vi "BStAT_(Singles).vi"() -> ()   [LabVIEW 2013]
uses:
  <vilib>/Utility/file.llb/Read From Spreadsheet File (DBL).vi
  <vilib>/Utility/file.llb/Write To Spreadsheet File (I64).vi
panel:
  out "framesPerSecond":u32
  out "serve to point":dbl[](array[numeric])
  in  "Word._Application":refnum<k7>
  out "p2y":dbl[](array[numeric])
  out "p1y":dbl[](array[numeric])
  out "point frames":dbl[](array[numeric])
  out "service frames":dbl[](array[numeric])
  out "comp_p1 2":dbl[](array[numeric])
  out "comp_p2 2":dbl[](array[numeric])
  out "comp_p2":dbl[](array[numeric])
  out "comp_p1":dbl[](array[numeric])
  out "game":i32[][](array[numeric])
  out "save2_data":dbl[][](array[numeric])
  out "save1_data":dbl[][](array[numeric])
  out "save2":i32[][](array[numeric])
  out "save1":i32[][](array[numeric])
  out "filedata in":dbl[][](array[numeric]) format="%0.3f"
  out "edited\nevents":dbl[][](array[numeric])
  out "edited to play":dbl[](array[numeric])
  out "P2 position":bool
  out "P1 position":bool
  out "p2code":i32
  out "p1code":i32
  out "frames":dbl[](array[numeric])
  out "Events":bool[](array[boolean])
  out "coded data":dbl[][](array[numeric])
  out "frame data":dbl[][](array[numeric])
  out "Score":dbl[][](array[numeric])
  out "OH":bool[](array[boolean])
  out "BH":bool[](array[boolean])
  out "FH":bool[](array[boolean])
  in  "stop":bool
  in  "Tab Control":enum32{"Coding", "Display"}(tab)
  in  "switch sides":bool
  in  "Drag control":u32(slide) min=400 max=3000 scale=0.0..6657.0
  in  "UNDO":bool
  out "Last coded":i32
  in  "Progress...":i32(slide) min=400 max=3000 scale=0.0..6657.0
  in  "1":bool
  in  "E2":bool
  in  "E1":bool
  in  "P2":i32
  in  "W2":bool
  in  "W1":bool
  in  "P1":i32
  in  "Pause 2":bool
  in  "F_Fr":bool
  in  "S_Fr":bool
  out "Video":T1(plugin-control)
  in  "START":bool
  in  "Video file":path caption="Open AVI file"
  in  "Save data":path caption="Save data to file"
  in  "Start Coding":bool
  out "F_frame":u32
  out "S_frame":u32
  in  "playback speed":dbl(slide) step=0.25 scale=0.25..2.0
  in  "fast forward":bool
  in  "TL 2":bool
  in  "BR 2":bool
  in  "BL 2":bool
  in  "BC 2":bool
  in  "MR  2":bool
  in  "MC 2":bool
  in  "ML 2":bool
  in  "TR 2":bool
  in  "TC 2":bool
  in  "TL 3":bool
  in  "BR 3":bool
  in  "BL 3":bool
  in  "BC 3":bool
  in  "MR  3":bool
  in  "MC 3":bool
  in  "ML 3":bool
  in  "TR 3":bool
  in  "TC 3":bool
  in  "Pause 1":bool
  out "coding":i32[][](array[numeric])
  in  "1 6":bool
  in  "2 6":bool
  in  "3 6":bool
  in  "4 6":bool
  in  "5 6":bool
  in  "6 6":bool
  in  "7 6":bool
  in  "8 6":bool
  in  "1 5":bool
  in  "2 5":bool
  in  "3 5":bool
  in  "4 5":bool
  in  "5 5":bool
  in  "6 5":bool
  in  "7 5":bool
  in  "8 5":bool
  in  "8 3":bool
  in  "7 3":bool
  in  "6 3":bool
  in  "5 3":bool
  in  "4 3":bool
  in  "3 3":bool
  in  "2 3":bool
  in  "1 3":bool
  in  "8 4":bool
  in  "7 4":bool
  in  "6 4":bool
  in  "5 4":bool
  in  "4 4":bool
  in  "3 4":bool
  in  "2 4":bool
  in  "1 4":bool
  in  "1 2":bool
  in  "2 2":bool
  in  "3 2":bool
  in  "4 2":bool
  in  "5 2":bool
  in  "6 2":bool
  in  "7 2":bool
  in  "8 2":bool
  in  "5":bool
  in  "6":bool
  in  "7":bool
  in  "8":bool
  in  "1":bool
  in  "2":bool
  in  "3":bool
  in  "4":bool
  in  "S2":bool
  in  "S1":bool
  in  "2":bool
  in  "3":bool
  in  "4":bool
  in  "Pause 3":bool
  in  "Stop and save":bool
  out "Numeric":dbl format="%<%H:%M:%S>t"
  in  "play back":i32(slide)=1 min=0 max=5284 scale=0.0..5284.0
  out "DISP":T1(plugin-control)
  in  "Vid file":path caption="Open AVI file"
  in  "Data file":path caption="Read data from"
  in  "Tab Control 2":enum32{"Edit ", "Data Display", "Momentum"}(tab)
  in  "shots":u8(slide)=2 scale=0.0..5.0
  in  "point 2":bool
  in  "Rally":bool
  in  "Write VI":path caption="Write to AVI file"
  in  "before":u8(slide)=2
  in  "Playback Speed":dbl(slide)=1.0 min=0.25 max=30.0 step=0.25 scale=0.25..2.0
  in  "pause":bool
  in  "stop 2":bool
  in  "Playback\nscore":bool
  in  "P2 score":dbl
  in  "P1 score":dbl
  in  "error":bool
  in  "winner":bool
  in  "point 1":bool
  in  "player1":bool
  in  "player2":bool
  in  "1 7":bool
  in  "service2":bool
  in  "service1":bool
  in  "2 7":bool
  in  "3 7":bool
  in  "4 7":bool
  in  "TL":bool
  in  "BR":bool
  in  "BL":bool
  in  "BM":bool
  in  "CR":bool
  in  "CM":bool
  in  "CL":bool
  in  "TR":bool
  in  "TM":bool
  in  "FH 2":bool
  in  "BH 2":bool
  in  "ST":bool
  in  "CR 2":bool
  in  "lob":bool
  in  "clear":bool
  in  "drive":bool
  in  "smash":bool
  in  "defense":bool
  in  "chop":bool
  in  "drop":bool
  in  "net":bool
  in  "OH 2":bool
  in  "Play":bool
  in  "after":u8(slide)=2 scale=0.0..5.0
  in  "write file":bool
  out "Search events":i32(slide) caption="Scaning(events)..." min=400 max=3000 scale=0.0..425.0
  out "Search score":i32(slide) caption="Searching(score)..." min=400 max=3000 scale=0.0..389.0
  out "writing":i32(slide) caption="Writing..." min=400 max=3000 scale=0.0..5284.0
  in  "3 shots":bool
  in  "Compare":bool
  in  "2":string(combo)="1"
  in  "1":string(combo)="1"
  in  "save2":string
  in  "save1":string
  in  "save2":bool
  in  "save1":bool
  in  "Percentage":bool
  in  "display\nselection":string(combo)="1"
  in  "To make white":enum32{""}(tab)
  out "player1 2":string[](array[string])
  out "player2 2":string[](array[string])
  out "P1graph":cluster{dbl[], "array":dbl[]}(graph)={[0.0, nan, 0.0, nan, 0.0, nan, 0.0, nan, 0.0, nan, 0.0, nan, 0.0, nan, 0.0, nan, 0.0], "array"=[1.0, 2.0, 3.0, 4.0, 5.0, 6.0, 7.0, 8.0, 9.0, 10.0, 11.0, 12.0, 13.0, 14.0, 15.0, 16.0, 17.0]}
  out "P2graph":cluster{dbl[], "array":dbl[]}(graph)={[0.0, nan, 0.0, nan, 0.0, nan, 0.0, nan, 0.0, nan, 0.0, nan, 0.0, nan, 0.0, nan, 0.0], "array"=[1.0, 2.0, 3.0, 4.0, 5.0, 6.0, 7.0, 8.0, 9.0, 10.0, 11.0, 12.0, 13.0, 14.0, 15.0, 16.0, 17.0]}
  out "W1/E1":string[](array[string])
  out "W2/E2":string[](array[string])
  out "W/E2":string[](array[string])=["Fore hand", "Back hand", "Over head", "", "Strainght", "Cross", "", "Lob", "Clear", "Drive", "Smash", "Defence", "Chop", "Drop", "Net"]
  out "W/E1":string[](array[string])=["Fore hand", "Back hand", "Over head", "", "Strainght", "Cross", "", "Lob", "Clear", "Drive", "Smash", "Defence", "Chop", "Drop", "Net"]
  out "player2_2":string[](array[string])
  out "player1_2":string[](array[string])
  out "Player 2":string[](array[string])=["Fore hand", "Back hand", "Over head", "", "Straight", "Cross", "", "Smash", "Defense", "Drive/Tap", "Lob", "Drop", "Chop", "Clear", "Net"]
  out "Player 2_2":string[](array[string])=["Fore hand", "Back hand", "Over head", "", "Strainght", "Cross", "", "Lob", "Clear", "Drive", "Smash", "Defence", "Chop", "Drop", "Net"]
  out "Player 1_2":string[](array[string])=["Fore hand", "Back hand", "Over head", "", "Strainght", "Cross", "", "Lob", "Clear", "Drive", "Smash", "Defence", "Chop", "Drop", "Net"]
  out "Player 1":string[](array[string])=["Fore hand", "Back hand", "Over head", "", "Straight", "Cross", "", "Smash", "Defense", "Drive/Tap", "Lob", "Drop", "Chop", "Clear", "Net"]
  out "p2 17":string
  out "p2 16":string
  out "p2 11":string
  out "p2 10":string
  out "p2 9":string
  out "p2 14":string
  out "p2 13":string
  out "p2 12":string
  out "p2 15":string
  out "p1 5":string
  out "p1 7":string
  out "p1 6":string
  out "p1 4":string
  out "p1 1":string
  out "p1 3":string
  out "p1 2":string
  out "p1 8":string
  out "p1 9":string
  in  "to make white 2":enum32{""}(tab)
  out "Shortest rally length(sec)":dbl format="%#_3g"
  out "Longest rally length(sec)":dbl format="%#_3g"
  out "momentum graph":cluster{dbl[], dbl[]}[](graph)
  out "Score":dbl[](array[numeric])
  out "Average rally length(sec)":dbl format="%#_3g"
  out "Rally length(sec)":dbl format="%#_3g"
  in  "edit video":bool
  in  "REPORT":bool
  # "Strategic Analysis Tool for Badminton"
  # "Forehand"
  # "Backhand"
  # "Overhead"
  # "Position"
  # "Straight"
  # "Cross"
  # "Straight"
  # "Cross"
  # "Straight"
  # "Cross"
  # "Smash"
  # "Defence"
  # "Drive/Tap"
  # "Lob"
  # "Drop"
  # "Chop"
  # "Clear"
  # "Net"
  # "Score"
  # "© 2014 National Sports Institute of Malaysia All Rights Reserved"
  # "© 2012 National Sports Institute of Malaysia All Rights Reserved"
  # "Shots to Playback"
  # "Score"
  # "Player"
  # "Position"
  # "Special Events"
  # "Playback interval (s)"
  # "to"
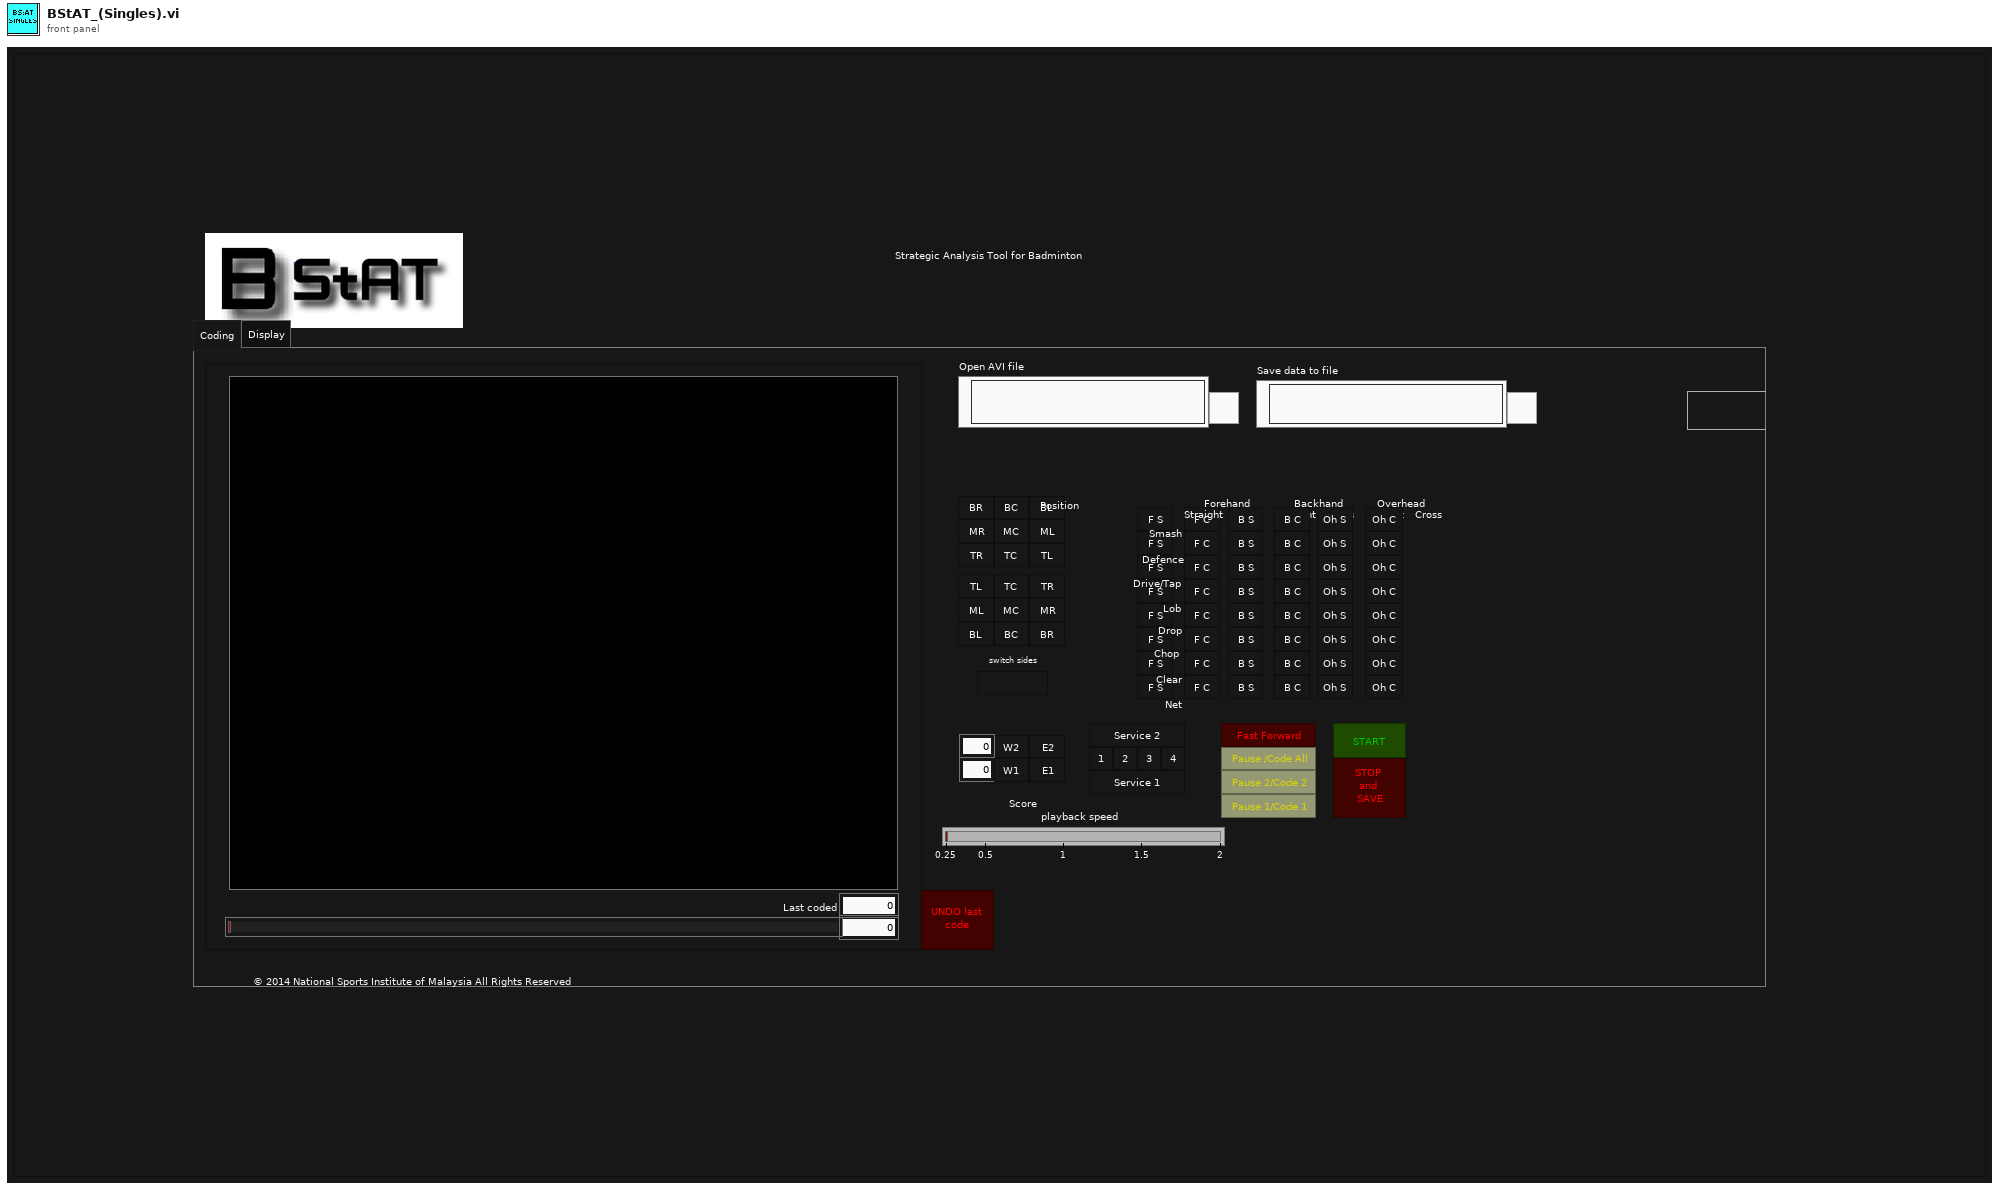
[diagram p1: front panel]
types:
  T1 = typedef "IMAQ Image.ctl" = refnum<image>
  T2 = enum8{"Enabled", "Disabled", "Disabled and Grayed Out"}
  T3 = enum16{"open", "replace", "create", "open or create", "replace or create", "replace or create with confirmation"}
  T4 = typedef "Image Type" = u32
  T5 = typedef "AviRefnum.ctl" = refnum<k1>
  T6 = cluster{"width":u32, "height":u32, "framesPerSecond":u32, "compressionFilter":string, "hasData":bool}
  T7 = typedef "LVPositionTypeDef.ctl" = cluster{"Left":i32, "Top":i32}
  T8 = cluster{"Position":T7, "Position":T7, "Position":T7, "Position":T7, "Position":T7, "Position":T7, "Position":T7, "Position":T7, "Position":T7, "Position":T7}
  T9 = cluster{"Position":T7, "Position":T7, "Position":T7, "Position":T7, "Position":T7, "Position":T7}
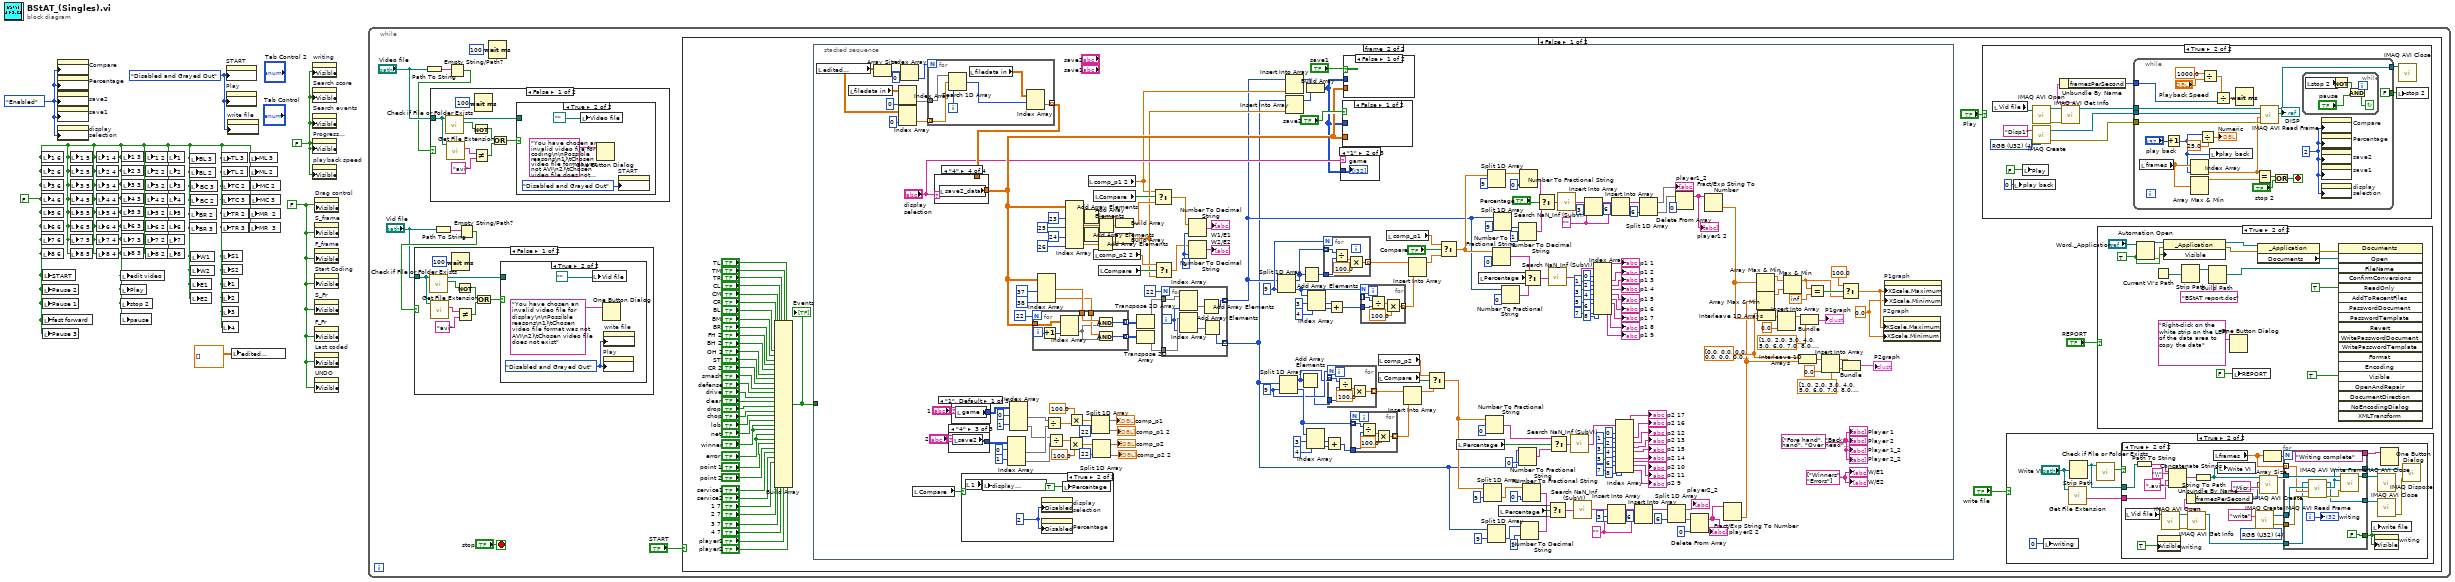
[diagram p0: block diagram]
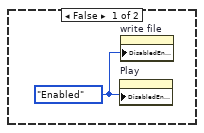
[diagram p2: hidden frame]
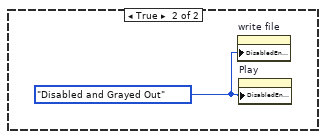
[diagram p3: hidden frame]
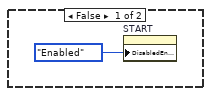
[diagram p4: hidden frame]
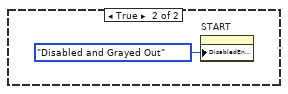
[diagram p5: hidden frame]
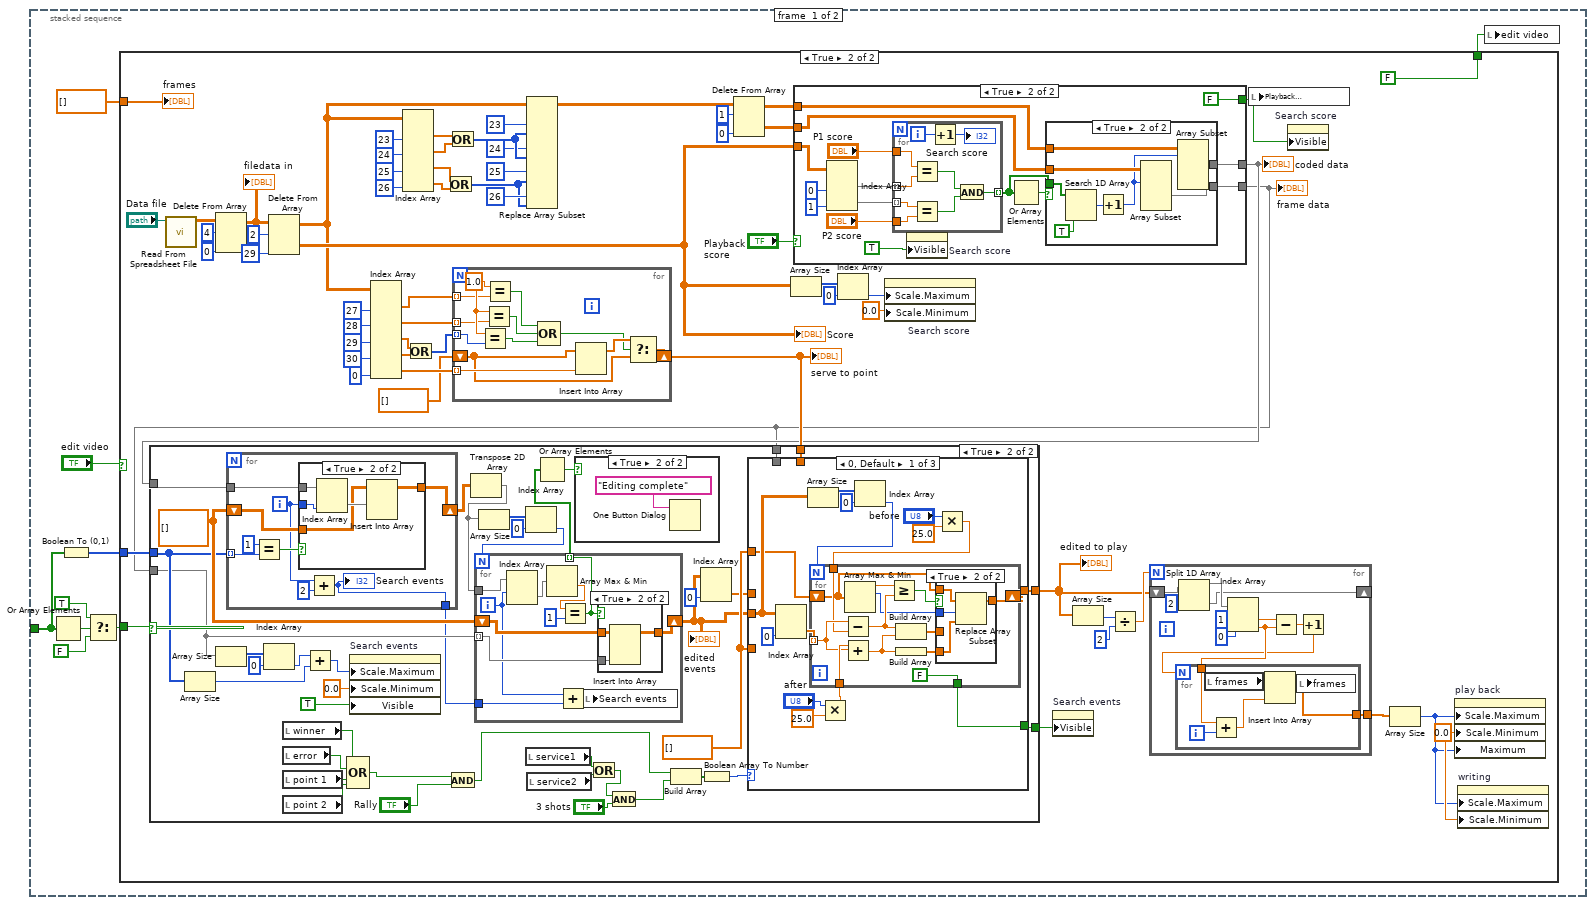
[diagram p7: hidden frame]
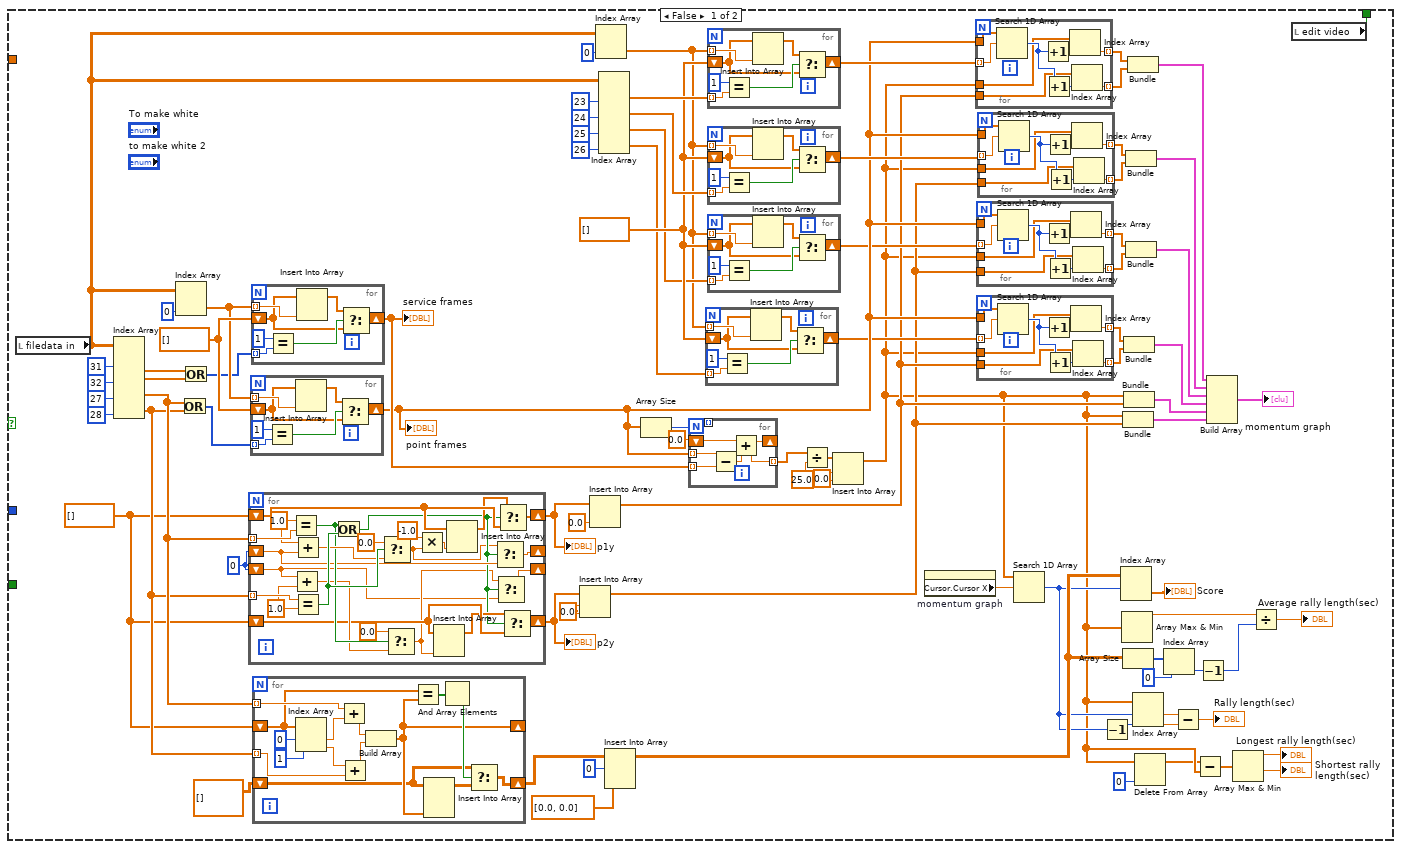
[diagram p8: hidden frame]
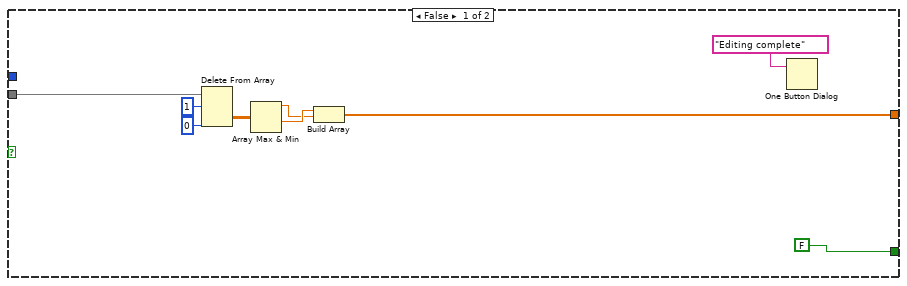
[diagram p9: hidden frame]
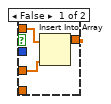
[diagram p10: hidden frame]
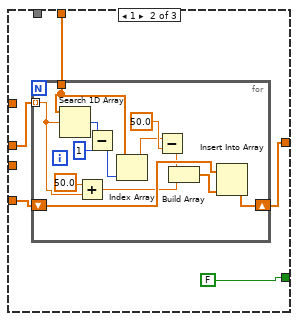
[diagram p11: hidden frame]
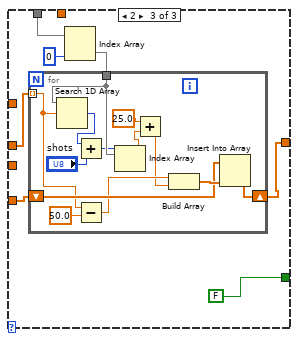
[diagram p12: hidden frame]
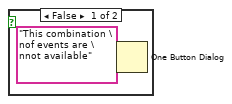
[diagram p13: hidden frame]
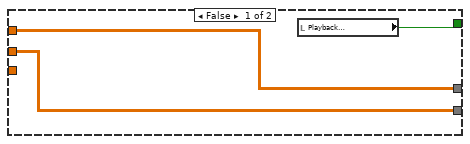
[diagram p16: hidden frame]
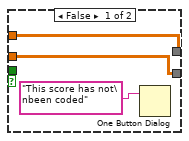
[diagram p17: hidden frame]
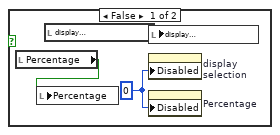
[diagram p18: hidden frame]
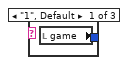
[diagram p19: hidden frame]
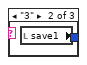
[diagram p20: hidden frame]
diagram:
  w1 = T2."Enabled" ("Disabled")
  w2 = T2."Disabled and Grayed Out" ("Disabled")
  w4 = FALSE ("4 6")
  w3 = FALSE ("Visible")
  w5 = FALSE ("Visible")
  n1 = local write "1 6"(w4) -> ()
  n2 = local write "2 6"(w4) -> ()
  n3 = local write "3 6"(w4) -> ()
  n4 = local write "4 6"(w4) -> ()
  n5 = local write "5 6"(w4) -> ()
  n6 = local write "6 6"(w4) -> ()
  n7 = local write "7 6"(w4) -> ()
  n8 = local write "8 6"(w4) -> ()
  n9 = local write "START"(w4) -> ()
  n10 = local write "Pause 2"(w4) -> ()
  n11 = local write "Pause 1"(w4) -> ()
  n12 = local write "fast forward"(w4) -> ()
  n13 = local write "Pause 3"(w4) -> ()
  n14 = property on="Compare" class="Bool (strict)"("DisabledEnum"=w1) -> ()  [unwired: 2 in, 2 out]
  n15 = property on="Percentage" class="Bool (strict)"("DisabledEnum"=w1) -> ()  [unwired: 2 in, 2 out]
  n16 = property on="save2" class="Bool (strict)"("DisabledEnum"=w1) -> ()  [unwired: 2 in, 2 out]
  n17 = property on="save1" class="Bool (strict)"("DisabledEnum"=w1) -> ()  [unwired: 2 in, 2 out]
  n18 = property on="display\nselection" class="CmbBox"("DisabledEnum"=w1) -> ()  [unwired: 2 in, 2 out]
  n19 = local write "1 5"(w4) -> ()
  n20 = local write "2 5"(w4) -> ()
  n21 = local write "3 5"(w4) -> ()
  n22 = local write "4 5"(w4) -> ()
  n23 = local write "5 5"(w4) -> ()
  n24 = local write "6 5"(w4) -> ()
  n25 = local write "7 5"(w4) -> ()
  n26 = local write "8 5"(w4) -> ()
  n27 = local write "1 4"(w4) -> ()
  n28 = local write "2 4"(w4) -> ()
  n29 = local write "3 4"(w4) -> ()
  n30 = local write "4 4"(w4) -> ()
  n31 = local write "5 4"(w4) -> ()
  n32 = local write "6 4"(w4) -> ()
  n33 = local write "7 4"(w4) -> ()
  n34 = local write "8 4"(w4) -> ()
  n35 = local write "edit video"(w4) -> ()
  n36 = local write "Play"(w4) -> ()
  n37 = local write "stop 2"(w4) -> ()
  n38 = local write "pause"(w4) -> ()
  n39 = local write "1 3"(w4) -> ()
  n40 = local write "2 3"(w4) -> ()
  n41 = local write "3 3"(w4) -> ()
  n42 = local write "4 3"(w4) -> ()
  n43 = local write "5 3"(w4) -> ()
  n44 = local write "6 3"(w4) -> ()
  n45 = local write "7 3"(w4) -> ()
  n46 = local write "8 3"(w4) -> ()
  n47 = local write "1 2"(w4) -> ()
  n48 = local write "2 2"(w4) -> ()
  n49 = local write "3 2"(w4) -> ()
  n50 = local write "4 2"(w4) -> ()
  n51 = local write "5 2"(w4) -> ()
  n52 = local write "6 2"(w4) -> ()
  n53 = local write "7 2"(w4) -> ()
  n54 = local write "8 2"(w4) -> ()
  n55 = local write "1"(w4) -> ()
  n56 = local write "2"(w4) -> ()
  n57 = local write "3"(w4) -> ()
  n58 = local write "4"(w4) -> ()
  n59 = local write "5"(w4) -> ()
  n60 = local write "6"(w4) -> ()
  n61 = local write "7"(w4) -> ()
  n62 = local write "8"(w4) -> ()
  n63 = local write "BL 3"(w4) -> ()
  n64 = local write "BL 2"(w4) -> ()
  n65 = local write "BR 2"(w4) -> ()
  n66 = local write "BR 3"(w4) -> ()
  n67 = local write "BC 3"(w4) -> ()
  n68 = local write "BC 2"(w4) -> ()
  n69 = local write "W1"(w4) -> ()
  n70 = local write "W2"(w4) -> ()
  n71 = local write "E1"(w4) -> ()
  n72 = local write "E2"(w4) -> ()
  n73 = local write "TL 3"(w4) -> ()
  n74 = local write "TL 2"(w4) -> ()
  n75 = local write "TR 2"(w4) -> ()
  n76 = local write "TR 3"(w4) -> ()
  n77 = local write "TC 2"(w4) -> ()
  n78 = local write "TC 3"(w4) -> ()
  n79 = local write "S1"(w4) -> ()
  n80 = local write "S2"(w4) -> ()
  n81 = local write "1"(w4) -> ()
  n82 = local write "2"(w4) -> ()
  n83 = local write "3"(w4) -> ()
  n84 = local write "4"(w4) -> ()
  n85 = property on="START" class="Bool (strict)"("DisabledEnum"=w2) -> ()  [unwired: 2 in, 2 out]
  n86 = property on="Play" class="Bool (strict)"("DisabledEnum"=w2) -> ()  [unwired: 2 in, 2 out]
  n87 = property on="write file" class="Bool (strict)"("DisabledEnum"=w2) -> ()  [unwired: 2 in, 2 out]
  n88 = local write "edited\nevents"(dbl[][] []) -> ()
  n89 = local write "ML 3"(w4) -> ()
  n90 = local write "ML 2"(w4) -> ()
  n91 = local write "MR  2"(w4) -> ()
  n92 = local write "MR  3"(w4) -> ()
  n93 = local write "MC 2"(w4) -> ()
  n94 = local write "MC 3"(w4) -> ()
  n95 = property on="writing" class="Slide (strict)"("Visible"=w5) -> ()  [unwired: 2 in, 2 out]
  n96 = property on="Search score" class="Slide (strict)"("Visible"=w5) -> ()  [unwired: 2 in, 2 out]
  n97 = property on="Search events" class="Slide (strict)"("Visible"=w5) -> ()  [unwired: 2 in, 2 out]
  n98 = property on="Progress..." class="Slide (strict)"("Visible"=w5) -> ()  [unwired: 2 in, 2 out]
  n99 = property on="playback speed" class="Slide (strict)"("Visible"=w5) -> ()  [unwired: 2 in, 2 out]
  n100 = property on="Drag control" class="Slide (strict)"("Visible"=w3) -> ()  [unwired: 2 in, 2 out]
  n101 = property on="S_frame" class="DigNum (strict)"("Visible"=w3) -> ()  [unwired: 2 in, 2 out]
  n102 = property on="F_frame" class="DigNum (strict)"("Visible"=w3) -> ()  [unwired: 2 in, 2 out]
  n103 = property on="Start Coding" class="Bool (strict)"("Visible"=w3) -> ()  [unwired: 2 in, 2 out]
  n104 = property on="S_Fr" class="Bool (strict)"("Visible"=w3) -> ()  [unwired: 2 in, 2 out]
  n105 = property on="F_Fr" class="Bool (strict)"("Visible"=w3) -> ()  [unwired: 2 in, 2 out]
  n106 = property on="Last coded" class="DigNum (strict)"("Visible"=w3) -> ()  [unwired: 2 in, 2 out]
  n107 = property on="UNDO" class="Bool (strict)"("Visible"=w3) -> ()  [unwired: 2 in, 2 out]
  n108 = while {
    stop <- "stop" stop-if-true
    n109 = Path To String(path="Video file") -> (string=w12:string)
    n110 = Path To String(path="Vid file") -> (string=w9:string)
    n111 = Empty String/Path?(string/path=w12) -> (empty?=w10:bool)
    n112 = case shown="False" w10 {
      tunnel: "Video file" -> [w38 _]
      frame False {
        n113 = call <vilib>:"Check if File or Folder Exists.vi"("path"=w38) -> ("file or folder exists?"=w33:bool, "dup path"=w34:path)  [unwired: 8 in, 1 out]
        n114 = call <vilib>:"Get File Extension.vi"("file"=w38) -> ("lowercase file extension"=w37:string)  [unwired: 7 in, 3 out]
        n115 = Not(x=w33) -> (.not. x?=w32:bool)
        n116 = Not Equal?(x=w37, y="avi" ("lowercase file extension")) -> (x != y?=w36:bool)
        n117 = Wait (ms)(milliseconds to wait=u32 100) -> ()  [unwired: 1 out]
        n118 = Or(x=w32, y=w36) -> (x .or. y?=w35:bool)
        n119 = case shown="True" w35 {
          tunnel: w34 -> [_ _]
          frame False {
            n120 = property on="START" class="Bool (strict)"("DisabledEnum"=T2."Enabled" ("Disabled")) -> ()  [unwired: 2 in, 2 out]
          }
          frame True {
            n121 = local write "Video file"(path "" ("Video file")) -> ()
            n122 = One Button Dialog(message="You have chosen an invalid video file for coding\n\nPossible reasons\n1)\tChosen video file format was not AVI\n2)\tChosen video file does not exist") -> ()  [unwired: 1 in, 1 out]
            n123 = property on="START" class="Bool (strict)"("DisabledEnum"=T2."Disabled and Grayed Out" ("Disabled")) -> ()  [unwired: 2 in, 2 out]
          }
        }
      }
      frame True {
        n124 = property on="START" class="Bool (strict)"("DisabledEnum"=T2."Disabled and Grayed Out" ("Disabled")) -> ()  [unwired: 2 in, 2 out]
      }
    }
    n125 = Empty String/Path?(string/path=w9) -> (empty?=w8:bool)
    n126 = case shown="False" w8 {
      tunnel: "Vid file" -> [w24 _]
      frame False {
        n127 = call <vilib>:"Check if File or Folder Exists.vi"("path"=w24) -> ("file or folder exists?"=w18:bool, "dup path"=w19:path)  [unwired: 8 in, 1 out]
        n128 = call <vilib>:"Get File Extension.vi"("file"=w24) -> ("lowercase file extension"=w23:string)  [unwired: 7 in, 3 out]
        n129 = Wait (ms)(milliseconds to wait=u32 100) -> ()  [unwired: 1 out]
        n130 = Not(x=w18) -> (.not. x?=w17:bool)
        n131 = Not Equal?(x=w23, y="avi" ("lowercase file extension")) -> (x != y?=w21:bool)
        n132 = Or(x=w17, y=w21) -> (x .or. y?=w20:bool)
        n133 = case shown="True" w20 {
          tunnel: w19 -> [_ _]
          frame False {
            w25 = T2."Enabled" ("Disabled")
            n134 = property on="Play" class="Bool (strict)"("DisabledEnum"=w25) -> ()  [unwired: 2 in, 2 out]
            n135 = property on="write file" class="Bool (strict)"("DisabledEnum"=w25) -> ()  [unwired: 2 in, 2 out]
          }
          frame True {
            w27 = T2."Disabled and Grayed Out" ("Disabled")
            n136 = local write "Vid file"(path "" ("Video file")) -> ()
            n137 = One Button Dialog(message="You have chosen an invalid video file for display\n\nPossible reasons\n1)\tChosen video file format was not AVI\n2)\tChosen video file does not exist") -> ()  [unwired: 1 in, 1 out]
            n138 = property on="Play" class="Bool (strict)"("DisabledEnum"=w27) -> ()  [unwired: 2 in, 2 out]
            n139 = property on="write file" class="Bool (strict)"("DisabledEnum"=w27) -> ()  [unwired: 2 in, 2 out]
          }
        }
      }
      frame True {
        w29 = T2."Disabled and Grayed Out" ("Disabled")
        n140 = property on="write file" class="Bool (strict)"("DisabledEnum"=w29) -> ()  [unwired: 2 in, 2 out]
        n141 = property on="Play" class="Bool (strict)"("DisabledEnum"=w29) -> ()  [unwired: 2 in, 2 out]
      }
    }
    n142 = Wait (ms)(milliseconds to wait=u32 100) -> ()  [unwired: 1 out]
    n143 = case shown="False" "START" {
      frame False {
        n144 = Build Array("TL", "TM", "TR", "CL", "CM", "CR", "BL", "BM", "BR", "FH 2", "BH 2", "OH 2", "ST", "CR 2", "smash", "defense", "drive", "clear", "drop", "chop", "lob", "net", "winner", "winner", "error", "error", "point 1", "point 2", "service1", "service2", "1 7", "2 7", "3 7", "4 7", "player1", "player2") -> (w56:bool[])
        "Events" <- w56
        n145 = stacked-sequence {
          tunnel: w56 -> [w103 _]
          frame #0 {
            n146 = Or Array Elements(Boolean array=w103) -> (logical OR=w106:bool)
            n147 = Boolean To (0,1)(Boolean=w103) -> (0, 1=w102:i16[])
            n148 = Select(t=TRUE, s=w106, f=FALSE) -> (s? t:f=w101:bool)
            n149 = case shown="True" "edit video" {
              tunnel: [w191 FALSE ("edit video")] -> w98
              tunnel: w102 -> [_ w320]
              tunnel: w101 -> [_ w359]
              tunnel: dbl[] [] ("edited\nto play 3") -> [_ w357]
              frame False {
                w147 = dbl[] []
                w181 = 0.0 ("new element/subarray")
                w180 = 0.0 ("new element/subarray")
                w179 = 0.0 ("new element/subarray")
                w129 = dbl[] []
                w132 = 0 ("disabled index (col)")
                w172 = dbl[] []
                n150 = local read "filedata in"() -> (w148:dbl[][])
                n151 = Index Array(array=w148, index (col) #1=31 ("length"), index (col) #2=32 ("disabled index (col)"), index (col) #3=27 ("index (col)"), index (col) #4=28 ("index (col)")) -> (element #1=w164:dbl[], element #2=w165:dbl[], element #3=w131:dbl[], element #4=w130:dbl[])  [unwired: 4 in]
                n152 = Index Array(array=w148, index (col)=0 ("disabled index (col)")) -> (element=w171:dbl[])  [unwired: 1 in]
                n153 = Or(x=w131, y=w130) -> (x .or. y?=w170:i32[])
                n154 = Or(x=w164, y=w165) -> (x .or. y?=w167:i32[])
                n155 = for {
                  shift-right: [w200] -> _
                  shift-left: w132 -> [w199]
                  shift-right: [w196] -> _
                  shift-left: w132 -> [w195]
                  shift-right: [w205] -> w127
                  shift-left: w129 -> [w204]
                  shift-right: [w211] -> w128
                  shift-left: w129 -> [w202]
                  tunnel: w130 -> [w208] mode=indexing
                  tunnel: w131 -> [w216] mode=indexing
                  w207 = 1.0 ("x")
                  w213 = 1.0 ("x")
                  n156 = Equal?(x=w213, y=w216) -> (x = y?=w209:bool)
                  n157 = Add(x=w195, y=w207) -> (x+y=w206:dbl)
                  n158 = Add(x=w213, y=w199) -> (x+y=w212:dbl)
                  n159 = Equal?(x=w208, y=w207) -> (x = y?=w215:bool)
                  n160 = Or(x=w209, y=w215) -> (x .or. y?=w198:bool)
                  n161 = Select(t=0.0, s=w215, f=w212) -> (s? t:f=w192:dbl)
                  n162 = Select(t=0.0, s=w209, f=w206) -> (s? t:f=w197:dbl)
                  n163 = Multiply(x=-1.0 ("y"), y=w192) -> (x*y=w194:dbl)
                  n164 = Insert Into Array(array=w202, new element=w197) -> (w201:dbl[])  [unwired: 1 in]
                  n165 = Insert Into Array(array=w204, new element=w194) -> (w203:dbl[])  [unwired: 1 in]
                  n166 = Select(t=w192, s=w198, f=w199) -> (s? t:f=w200:dbl)
                  n167 = Select(t=w197, s=w198, f=w195) -> (s? t:f=w196:dbl)
                  n168 = Select(t=w203, s=w198, f=w204) -> (s? t:f=w205:dbl[])
                  n169 = Select(t=w201, s=w198, f=w202) -> (s? t:f=w211:dbl[])
                }
                "p1y" <- w127
                "p2y" <- w128
                n170 = for {
                  tunnel: w170 -> [w308] mode=indexing
                  tunnel: w171 -> [w304] mode=indexing
                  shift-right: [w303] -> w143
                  shift-left: w172 -> [w302]
                  n171 = Equal?(x=1, y=w308) -> (x = y?=w306:bool)
                  n172 = Insert Into Array(array=w302, new element=w304) -> (w305:dbl[])  [unwired: 1 in]
                  n173 = Select(t=w305, s=w306, f=w302) -> (s? t:f=w303:dbl[])
                }
                "point frames" <- w143
                n174 = for {
                  tunnel: w167 -> [w315] mode=indexing
                  tunnel: w171 -> [w311] mode=indexing
                  shift-right: [w310] -> w174
                  shift-left: w172 -> [w309]
                  n175 = Equal?(x=1, y=w315) -> (x = y?=w313:bool)
                  n176 = Insert Into Array(array=w309, new element=w311) -> (w312:dbl[])  [unwired: 1 in]
                  n177 = Select(t=w312, s=w313, f=w309) -> (s? t:f=w310:dbl[])
                }
                "service frames" <- w174
                n178 = for {
                  tunnel: w131 -> [w292] mode=indexing
                  tunnel: w130 -> [w288] mode=indexing
                  shift-right: [w284] -> _
                  shift-left: w129 -> [w287]
                  shift-right: [w282] -> w186
                  shift-left: dbl[][] [] -> [w281]
                  n179 = Index Array(array=w287, index #1=0 ("index"), index #2=1 ("index")) -> (element #1=w293:dbl, element #2=w291:dbl)
                  n180 = Add(x=w292, y=w293) -> (x+y=w290:dbl)
                  n181 = Add(x=w291, y=w288) -> (x+y=w289:dbl)
                  n182 = Build Array(w290, w289) -> (w284:dbl[])
                  n183 = Equal?(x=w287, y=w284) -> (x = y?=w286:bool[])
                  n184 = Insert Into Array(array=w281, new element=w284) -> (w283:dbl[][])  [unwired: 2 in]
                  n185 = And Array Elements(Boolean array=w286) -> (logical AND=w285:bool)
                  n186 = Select(t=w281, s=w285, f=w283) -> (s? t:f=w282:dbl[][])
                }
                n187 = Insert Into Array(array=w128, index=w180, new element=w180) -> (w125:dbl[])
                n188 = Insert Into Array(array=w127, index=w181, new element=w181) -> (w126:dbl[])
                n189 = Index Array(array=w148, index (col)=0 ("disabled index (col)")) -> (element=w144:dbl[])  [unwired: 1 in]
                n190 = Index Array(array=w148, index (col) #1=23 ("disabled index (col)"), index (col) #2=24 ("index (col)"), index (col) #3=25 ("index (col)"), index (col) #4=26 ("index (col)")) -> (element #1=w157:dbl[], element #2=w158:dbl[], element #3=w146:dbl[], element #4=w145:dbl[])  [unwired: 4 in]
                n191 = Insert Into Array(array=w186, index (row)=0, new element=dbl[] [0.0, 0.0] ("new element/subarray")) -> (w124:dbl[][])  [unwired: 1 in]
                n192 = Array Size(array=w143) -> (size(s)=w173:i32)
                n193 = for {
                  N: w173 -> [w296]
                  tunnel: w143 -> [w301] mode=indexing
                  tunnel: w174 -> [w300] mode=indexing
                  tunnel: [w297] -> w183 mode=indexing
                  shift-right: [w297] -> _
                  shift-left: 0.0 -> [w298]
                  tunnel: [w296] -> _ mode=indexing
                  n194 = Subtract(x=w301, y=w300) -> (x-y=w299:dbl)
                  n195 = Add(x=w298, y=w299) -> (x+y=w297:dbl)
                }
                n196 = for {
                  tunnel: w145 -> [w241] mode=indexing
                  tunnel: w144 -> [w237] mode=indexing
                  shift-right: [w236] -> w141
                  shift-left: w147 -> [w235]
                  n197 = Equal?(x=1, y=w241) -> (x = y?=w239:bool)
                  n198 = Insert Into Array(array=w235, new element=w237) -> (w238:dbl[])  [unwired: 1 in]
                  n199 = Select(t=w238, s=w239, f=w235) -> (s? t:f=w236:dbl[])
                }
                n200 = for {
                  tunnel: w157 -> [w280] mode=indexing
                  tunnel: w144 -> [w276] mode=indexing
                  shift-right: [w275] -> w154
                  shift-left: w147 -> [w274]
                  n201 = Equal?(x=1, y=w280) -> (x = y?=w278:bool)
                  n202 = Insert Into Array(array=w274, new element=w276) -> (w277:dbl[])  [unwired: 1 in]
                  n203 = Select(t=w277, s=w278, f=w274) -> (s? t:f=w275:dbl[])
                }
                n204 = for {
                  tunnel: w158 -> [w273] mode=indexing
                  tunnel: w144 -> [w269] mode=indexing
                  shift-right: [w268] -> w159
                  shift-left: w147 -> [w267]
                  n205 = Equal?(x=1, y=w273) -> (x = y?=w271:bool)
                  n206 = Insert Into Array(array=w267, new element=w269) -> (w270:dbl[])  [unwired: 1 in]
                  n207 = Select(t=w270, s=w271, f=w267) -> (s? t:f=w268:dbl[])
                }
                n208 = for {
                  tunnel: w146 -> [w248] mode=indexing
                  tunnel: w144 -> [w244] mode=indexing
                  shift-right: [w243] -> w142
                  shift-left: w147 -> [w242]
                  n209 = Equal?(x=1, y=w248) -> (x = y?=w246:bool)
                  n210 = Insert Into Array(array=w242, new element=w244) -> (w245:dbl[])  [unwired: 1 in]
                  n211 = Select(t=w245, s=w246, f=w242) -> (s? t:f=w243:dbl[])
                }
                n212 = Divide(x=w183, y=25.0 ("new element/subarray")) -> (x/y=w182:dbl[])
                n213 = Insert Into Array(array=w182, index=w179, new element=w179) -> (w111:dbl[])
                n214 = property on="momentum graph" class="XYGraph (strict)"() -> ("Cursor.Cursor X"=w189:dbl)  [unwired: 2 in, 2 out]
                n215 = for {
                  tunnel: w154 -> [w266] mode=indexing
                  tunnel: w143 -> [w265]
                  tunnel: [w263] -> w155 mode=indexing
                  tunnel: [w260] -> w156 mode=indexing
                  tunnel: w111 -> [w259]
                  tunnel: w126 -> [w258]
                  n216 = Search 1D Array(1D array=w265, element=w266) -> (index of element=w261:i32)  [unwired: 1 in]
                  n217 = Increment(x=w261) -> (x+1=w264:i32)
                  n218 = Increment(x=w261) -> (x+1=w262:i32)
                  n219 = Index Array(array=w259, index=w264) -> (element=w263:dbl)
                  n220 = Index Array(array=w258, index=w262) -> (element=w260:dbl)
                }
                n221 = for {
                  tunnel: w142 -> [w234] mode=indexing
                  tunnel: w143 -> [w233]
                  tunnel: [w231] -> w140 mode=indexing
                  tunnel: [w228] -> w139 mode=indexing
                  tunnel: w111 -> [w227]
                  tunnel: w125 -> [w226]
                  n222 = Search 1D Array(1D array=w233, element=w234) -> (index of element=w229:i32)  [unwired: 1 in]
                  n223 = Increment(x=w229) -> (x+1=w232:i32)
                  n224 = Increment(x=w229) -> (x+1=w230:i32)
                  n225 = Index Array(array=w227, index=w232) -> (element=w231:dbl)
                  n226 = Index Array(array=w226, index=w230) -> (element=w228:dbl)
                }
                n227 = for {
                  tunnel: w141 -> [w225] mode=indexing
                  tunnel: w143 -> [w224]
                  tunnel: [w222] -> w138 mode=indexing
                  tunnel: [w219] -> w137 mode=indexing
                  tunnel: w111 -> [w218]
                  tunnel: w126 -> [w217]
                  n228 = Search 1D Array(1D array=w224, element=w225) -> (index of element=w220:i32)  [unwired: 1 in]
                  n229 = Increment(x=w220) -> (x+1=w223:i32)
                  n230 = Increment(x=w220) -> (x+1=w221:i32)
                  n231 = Index Array(array=w218, index=w223) -> (element=w222:dbl)
                  n232 = Index Array(array=w217, index=w221) -> (element=w219:dbl)
                }
                n233 = for {
                  tunnel: w159 -> [w257] mode=indexing
                  tunnel: w143 -> [w256]
                  tunnel: [w254] -> w160 mode=indexing
                  tunnel: [w251] -> w161 mode=indexing
                  tunnel: w111 -> [w250]
                  tunnel: w125 -> [w249]
                  n234 = Search 1D Array(1D array=w256, element=w257) -> (index of element=w252:i32)  [unwired: 1 in]
                  n235 = Increment(x=w252) -> (x+1=w255:i32)
                  n236 = Increment(x=w252) -> (x+1=w253:i32)
                  n237 = Index Array(array=w250, index=w255) -> (element=w254:dbl)
                  n238 = Index Array(array=w249, index=w253) -> (element=w251:dbl)
                }
                n239 = Search 1D Array(1D array=w111, element=w189) -> (index of element=w116:i32)  [unwired: 1 in]
                n240 = Decrement(x=w116) -> (x-1=w117:i32)
                n241 = Index Array(array=w124, index (row)=w116) -> (element=→"Score":dbl[])  [unwired: 1 in]
                n242 = Array Max & Min(array=w111) -> (max value=w120:dbl)  [unwired: 3 out]
                n243 = Bundle(w111, w125) -> (w175:cluster{dbl[], dbl[]})  [unwired: 1 in]
                n244 = Array Size(array=w124) -> (size(s)=w123:i32[])
                n245 = Bundle(w138, w137) -> (w133:cluster{dbl[], dbl[]})  [unwired: 1 in]
                n246 = Bundle(w111, w126) -> (w176:cluster{dbl[], dbl[]})  [unwired: 1 in]
                n247 = Bundle(w160, w161) -> (w135:cluster{dbl[], dbl[]})  [unwired: 1 in]
                n248 = Bundle(w140, w139) -> (w134:cluster{dbl[], dbl[]})  [unwired: 1 in]
                n249 = Bundle(w155, w156) -> (w136:cluster{dbl[], dbl[]})  [unwired: 1 in]
                n250 = Index Array(array=w111, index #1=w116, index #2=w117) -> (element #1=w114:dbl, element #2=w115:dbl)
                n251 = Delete From Array(array=w111, index=0) -> (array with subset deleted=w110:dbl[])  [unwired: 1 in, 1 out]
                n252 = Index Array(array=w123, index=0) -> (element=w121:i32)
                n253 = Subtract(x=w114, y=w115) -> (x-y=→"Rally length(sec)":dbl)
                n254 = Subtract(x=w110, y=w111) -> (x-y=w109:dbl[])
                n255 = Decrement(x=w121) -> (x-1=w119:i32)
                n256 = Build Array(w136, w135, w134, w133, w176, w175) -> (→"momentum graph":cluster{dbl[], dbl[]}[])
                n257 = Array Max & Min(array=w109) -> (max value=→"Longest rally length(sec)":dbl, min value=→"Shortest rally length(sec)":dbl)  [unwired: 2 out]
                n258 = Divide(x=w120, y=w119) -> (x/y=→"Average rally length(sec)":dbl)
                n259 = local read "edit video"() -> (w191:bool)
              }
              frame True {
                w355 = 0.0 ("Scale.Range:Minimum")
                n260 = call-poly <vilib>:"Read From Spreadsheet File.vi"("file path (dialog if empty)"="Data file") -> ("all rows"=w373:dbl[][])  [unwired: 6 in, 4 out]
                n261 = Delete From Array(array=w373, length=4, index (row)=0) -> (array with subset deleted=w352:dbl[][])  [unwired: 1 in, 1 out]
                "filedata in" <- w352
                n262 = Delete From Array(array=w352, length=2, index (col)=29 ("disabled index (col)")) -> (deleted portion=w364:dbl[][], array with subset deleted=w319:dbl[][])  [unwired: 1 in]
                "Score" <- w364
                n263 = Index Array(array=w319, index (col) #1=27 ("disabled index (col)"), index (col) #2=28 ("index (col)"), index (col) #3=29 ("index (col)"), index (col) #4=30 ("index (col)"), index (col) #5=0 ("index (col)")) -> (element #1=w326:dbl[], element #2=w327:dbl[], element #3=w325:dbl[], element #4=w324:dbl[], element #5=w329:dbl[])  [unwired: 5 in]
                n264 = Index Array(array=w319, index (col) #1=23 ("disabled index (col)"), index (col) #2=24 ("index (col)"), index (col) #3=25 ("index (col)"), index (col) #4=26 ("index (col)")) -> (element #1=w347:dbl[], element #2=w346:dbl[], element #3=w345:dbl[], element #4=w344:dbl[])  [unwired: 4 in]
                n265 = Or(x=w325, y=w324) -> (x .or. y?=w328:i32[])
                n266 = Or(x=w345, y=w344) -> (x .or. y?=w338:i32[])
                n267 = Or(x=w347, y=w346) -> (x .or. y?=w343:i32[])
                n268 = for {
                  tunnel: w326 -> [w379] mode=indexing
                  tunnel: w329 -> [w383] mode=indexing
                  tunnel: w328 -> [w377] mode=indexing
                  tunnel: w327 -> [w378] mode=indexing
                  shift-right: [w385] -> w323
                  shift-left: dbl[] [] -> [w382]
                  w384 = 1.0 ("x")
                  n269 = Equal?(x=w384, y=w377) -> (x = y?=w386:bool)
                  n270 = Equal?(x=w384, y=w378) -> (x = y?=w387:bool)
                  n271 = Equal?(x=w384, y=w379) -> (x = y?=w388:bool)
                  n272 = Compound Arithmetic op=OR(w388, w387, w386) -> (w380:bool)
                  n273 = Insert Into Array(array=w382, new element=w383) -> (w381:dbl[])  [unwired: 1 in]
                  n274 = Select(t=w381, s=w380, f=w382) -> (s? t:f=w385:dbl[])
                }
                "serve to point" <- w323
                n275 = Replace Array Subset(array=w319, new element #1=w343, index (col) #1=23 ("disabled index (col)"), new element #2=w343, index (col) #2=24 ("index (col)"), new element #3=w338, index (col) #3=25 ("index (col)"), new element #4=w338, index (col) #4=26 ("index (col)")) -> (w318:dbl[][])  [unwired: 4 in]
                n276 = Delete From Array(array=w318, length=1, index (col)=0 ("disabled index (col)")) -> (deleted portion=w367:dbl[][], array with subset deleted=w368:dbl[][])  [unwired: 1 in]
                n277 = Array Size(array=w364) -> (size(s)=w365:i32[])
                n278 = case shown="True" "Playback\nscore" {
                  tunnel: w368 -> [w561 w568]
                  tunnel: w367 -> [w560 w567]
                  tunnel: w364 -> [_ w577]
                  tunnel: [w562 FALSE ("element")] -> w361
                  tunnel: [w560 w565] -> w317
                  tunnel: [w561 w564] -> w322
                  frame False {
                    n279 = local read "Playback\nscore"() -> (w562:bool)
                  }
                  frame True {
                    n280 = Index Array(array=w577, index (col) #1=0 ("disabled index (col)"), index (col) #2=1 ("index (col)")) -> (element #1=w574:dbl[], element #2=w573:dbl[])  [unwired: 2 in]
                    n281 = for {
                      tunnel: w574 -> [w597] mode=indexing
                      tunnel: w573 -> [w595] mode=indexing
                      tunnel: "P1 score" -> [w596]
                      tunnel: "P2 score" -> [w594]
                      tunnel: [w592] -> w569 mode=indexing
                      i -> [w591]
                      n282 = Equal?(x=w596, y=w597) -> (x = y?=w593:bool)
                      n283 = Equal?(x=w595, y=w594) -> (x = y?=w589:bool)
                      n284 = Increment(x=w591) -> (x+1=→"Search score":i32)
                      n285 = And(x=w593, y=w589) -> (x .and. y?=w592:bool)
                    }
                    n286 = property on="Search score" class="Slide (strict)"("Visible"=TRUE) -> ()  [unwired: 2 in, 2 out]
                    n287 = Or Array Elements(Boolean array=w569) -> (logical OR=w570:bool)
                    n288 = case shown="True" w570 {
                      tunnel: w569 -> [_ w588]
                      tunnel: w568 -> [w580 w586]
                      tunnel: w567 -> [w579 w585]
                      tunnel: [w580 w584] -> w564
                      tunnel: [w579 w583] -> w565
                      frame False {
                        n289 = One Button Dialog(message="This score has not\nbeen coded") -> ()  [unwired: 1 in, 1 out]
                      }
                      frame True {
                        n290 = Search 1D Array(1D array=w588, element=TRUE) -> (index of element=w582:i32)  [unwired: 1 in]
                        n291 = Increment(x=w582) -> (x+1=w581:i32)
                        n292 = Array Subset(array=w585, index (row)=w581) -> (w583:dbl[][])  [unwired: 3 in]
                        n293 = Array Subset(array=w586, index (row)=w581) -> (w584:dbl[][])  [unwired: 3 in]
                      }
                    }
                  }
                }
                "frame data" <- w317
                "coded data" <- w322
                n294 = case shown="True" w359 {
                  tunnel: w322 -> [_ w454]
                  tunnel: w320 -> [_ w445]
                  tunnel: w317 -> [w408 w442]
                  tunnel: [w411 w435] -> w336
                  tunnel: [FALSE ("Visible") w434] -> w335
                  tunnel: w323 -> [_ w432]
                  tunnel: w317 -> [_ w428]
                  frame False {
                    n295 = Delete From Array(array=w408, length=1, index (col)=0 ("disabled index (col)")) -> (deleted portion=w407:dbl[][])  [unwired: 1 in, 1 out]
                    n296 = Array Max & Min(array=w407) -> (max value=w409:dbl, min value=w410:dbl)  [unwired: 2 out]
                    n297 = Build Array(w410, w409) -> (w411:dbl[])
                    n298 = One Button Dialog(message="Editing complete") -> ()  [unwired: 1 in, 1 out]
                  }
                  frame True {
                    w433 = dbl[] []
                    w446 = dbl[][] []
                    n299 = Array Size(array=w445) -> (size(s)=w439:i32)
                    n300 = Array Size(array=w442) -> (size(s)=w443:i32[])
                    n301 = for {
                      tunnel: w445 -> [w553] mode=indexing
                      tunnel: w454 -> [w550]
                      shift-right: [w549] -> w453
                      shift-left: w446 -> [w548]
                      tunnel: [w545] -> w437
                      i -> [w547]
                      n302 = Equal?(x=i16 1, y=w553) -> (x = y?=w551:bool)
                      n303 = case shown="True" w551 {
                        tunnel: w547 -> [_ w559]
                        tunnel: w550 -> [_ w558]
                        tunnel: [w554 w556] -> w549
                        tunnel: w548 -> [w554 w555]
                        frame False {
                        }
                        frame True {
                          n304 = Index Array(array=w558, index (col)=w559) -> (element=w557:dbl[])  [unwired: 1 in]
                          n305 = Insert Into Array(array=w555, new element=w557) -> (w556:dbl[][])  [unwired: 2 in]
                        }
                      }
                      n306 = Add(x=w547, y=2) -> (x+y=w545:i32)
                      "Search events" <- w545
                    }
                    n307 = Index Array(array=w443, index=0) -> (element=w438:i32)
                    n308 = local read "winner"() -> (w416:bool)
                    n309 = local read "error"() -> (w417:bool)
                    n310 = local read "point 1"() -> (w418:bool)
                    n311 = local read "point 2"() -> (w419:bool)
                    n312 = Add(x=w438, y=w439) -> (x+y=w441:i32)
                    n313 = Compound Arithmetic op=OR(w416, w417, w418, w419) -> (w415:bool)
                    n314 = property on="Search events" class="Slide (strict)"("Scale.Maximum"=w441, "Scale.Minimum"=0.0 ("Scale.Range:Minimum"), "Visible"=TRUE) -> ()  [unwired: 2 in, 2 out]
                    n315 = And(x=w415, y="Rally") -> (x .and. y?=w414:bool)
                    n316 = Transpose 2D Array(2D array=w453) -> (transposed array=w449:dbl[][])
                    n317 = Array Size(array=w449) -> (size(s)=w452:i32[])
                    n318 = Index Array(array=w452, index=0) -> (element=w450:i32)
                    n319 = for {
                      N: w450 -> [_]
                      tunnel: w442 -> [w538] mode=indexing
                      shift-right: [w537] -> w431
                      shift-left: w446 -> [w539]
                      tunnel: w449 -> [w536]
                      tunnel: [w533] -> w448 mode=indexing
                      tunnel: w437 -> [w530]
                      i -> [w531]
                      n320 = Index Array(array=w536, index (row)=w531) -> (element=w535:dbl[])  [unwired: 1 in]
                      n321 = Array Max & Min(array=w535) -> (min value=w534:dbl)  [unwired: 3 out]
                      n322 = Add(x=w531, y=w530) -> (x+y=w532:i32)
                      n323 = Equal?(x=w534, y=1) -> (x = y?=w533:bool)
                      n324 = local write "Search events"(w532) -> ()
                      n325 = case shown="True" w533 {
                        tunnel: w539 -> [w541 w544]
                        tunnel: w538 -> [_ w543]
                        tunnel: [w541 w542] -> w537
                        frame False {
                        }
                        frame True {
                          n326 = Insert Into Array(array=w544, new element=w543) -> (w542:dbl[][])  [unwired: 2 in]
                        }
                      }
                    }
                    "edited\nevents" <- w431
                    n327 = local read "service1"() -> (w422:bool)
                    n328 = local read "service2"() -> (w423:bool)
                    n329 = Or Array Elements(Boolean array=w448) -> (logical OR=w447:bool)
                    n330 = case shown="True" w447 {
                      frame False {
                        n331 = One Button Dialog(message="This combination \nof events are \nnot available") -> ()  [unwired: 1 in, 1 out]
                      }
                      frame True {
                        n332 = One Button Dialog(message="Editing complete") -> ()  [unwired: 1 in, 1 out]
                      }
                    }
                    n333 = Or(x=w422, y=w423) -> (x .or. y?=w425:bool)
                    n334 = And(x=w425, y="3 shots") -> (x .and. y?=w421:bool)
                    n335 = Build Array(w414, w421) -> (w427:bool[])
                    n336 = Index Array(array=w431, index (col)=0 ("disabled index (col)")) -> (element=w429:dbl[])  [unwired: 1 in]
                    n337 = Boolean Array To Number(Boolean array=w427) -> (number=w426:u32)
                    n338 = case shown="0, Default" w426 {
                      tunnel: w431 -> [w458 _ _]
                      tunnel: [w457 w492 w508] -> w435
                      tunnel: [w456 FALSE ("Visible") FALSE ("Visible")] -> w434
                      tunnel: w433 -> [w455 _ _]
                      tunnel: w433 -> [_ w494 w512]
                      tunnel: w432 -> [_ w493 _]
                      tunnel: w429 -> [_ w490 w513]
                      tunnel: w428 -> [_ _ w511]
                      frame 0, Default {
                        n339 = Index Array(array=w458, index (col)=0 ("disabled index (col)")) -> (element=w460:dbl[])  [unwired: 1 in]
                        n340 = Array Size(array=w458) -> (size(s)=w464:i32[])
                        n341 = Multiply(x="after", y=25.0) -> (x*y=w462:dbl)
                        n342 = Index Array(array=w464, index=0) -> (element=w459:i32)
                        n343 = Multiply(x="before", y=25.0) -> (x*y=w463:dbl)
                        n344 = for {
                          N: w459 -> [_]
                          tunnel: w463 -> [w480]
                          tunnel: w462 -> [w482]
                          tunnel: w460 -> [w481] mode=indexing
                          shift-right: [w472] -> w457
                          shift-left: w455 -> [w476]
                          tunnel: [FALSE ("Visible")] -> w456
                          n345 = Subtract(x=w481, y=w480) -> (x-y=w478:dbl)
                          n346 = Add(x=w482, y=w481) -> (x+y=w477:dbl)
                          n347 = Array Max & Min(array=w476) -> (max value=w479:dbl, max index (indices)=w474:i32)  [unwired: 2 out]
                          n348 = Greater Or Equal?(x=w479, y=w478) -> (x >= y?=w475:bool)
                          n349 = Build Array(w478, w477) -> (w471:dbl[])
                          n350 = Build Array(w477) -> (w473:dbl[])
                          n351 = case shown="True" w475 {
                            tunnel: w476 -> [w485 w489]
                            tunnel: w474 -> [_ w488]
                            tunnel: w473 -> [_ w487]
                            tunnel: [w484 w486] -> w472
                            tunnel: w471 -> [w483 _]
                            frame False {
                              n352 = Insert Into Array(array=w485, new element=w483) -> (w484:dbl[])  [unwired: 1 in]
                            }
                            frame True {
                              n353 = Replace Array Subset(array=w489, new element=w487, index=w488) -> (w486:dbl[])
                            }
                          }
                        }
                      }
                      frame 1 {
                        n354 = for {
                          tunnel: w490 -> [w495] mode=indexing
                          shift-right: [w502] -> w492
                          shift-left: w494 -> [w503]
                          tunnel: w493 -> [w496]
                          n355 = Search 1D Array(1D array=w496, element=w495) -> (index of element=w507:i32)  [unwired: 1 in]
                          n356 = Add(x=50.0, y=w495) -> (x+y=w500:dbl)
                          n357 = Subtract(x=w507, y=1) -> (x-y=w505:i32)
                          n358 = Index Array(array=w496, index=w505) -> (element=w497:dbl)
                          n359 = Subtract(x=w497, y=50.0 ("x")) -> (x-y=w501:dbl)
                          n360 = Build Array(w501, w500) -> (w504:dbl[])
                          n361 = Insert Into Array(array=w503, new element=w504) -> (w502:dbl[])  [unwired: 1 in]
                        }
                      }
                      frame 2 {
                        n362 = Index Array(array=w511, index (col)=0 ("disabled index (col)")) -> (element=w509:dbl[])  [unwired: 1 in]
                        n363 = for {
                          tunnel: w513 -> [w517] mode=indexing
                          shift-right: [w525] -> w508
                          shift-left: w512 -> [w526]
                          tunnel: w509 -> [w520]
                          n364 = Search 1D Array(1D array=w520, element=w517) -> (index of element=w519:i32)  [unwired: 1 in]
                          n365 = Add(x=w519, y="shots") -> (x+y=w518:i32)
                          n366 = Subtract(x=w517, y=50.0 ("x")) -> (x-y=w524:dbl)
                          n367 = Index Array(array=w520, index=w518) -> (element=w516:dbl)
                          n368 = Add(x=25.0, y=w516) -> (x+y=w523:dbl)
                          n369 = Build Array(w524, w523) -> (w527:dbl[])
                          n370 = Insert Into Array(array=w526, new element=w527) -> (w525:dbl[])  [unwired: 1 in]
                        }
                      }
                    }
                  }
                }
                "edited to play" <- w336
                n371 = Index Array(array=w365, index=0) -> (element=w363:i32)
                n372 = property on="Search score" class="Slide (strict)"("Scale.Maximum"=w363, "Scale.Minimum"=0.0 ("Scale.Range:Minimum")) -> ()  [unwired: 2 in, 2 out]
                n373 = property on="Search events" class="Slide (strict)"("Visible"=w335) -> ()  [unwired: 2 in, 2 out]
                n374 = Array Size(array=w336) -> (size(s)=w358:i32)
                n375 = Divide(x=w358, y=2) -> (x/y=w354:dbl)
                n376 = for {
                  N: w354 -> [_]
                  shift-right: [w393] -> _
                  shift-left: w336 -> [w395]
                  tunnel: [w389] -> w356
                  n377 = Split 1D Array(array=w395, index=2) -> (first subarray=w394:dbl[], second subarray=w393:dbl[])
                  n378 = Index Array(array=w394, index #1=1 ("index"), index #2=0 ("index")) -> (element #1=w399:dbl, element #2=w392:dbl)
                  n379 = Subtract(x=w399, y=w392) -> (x-y=w391:dbl)
                  n380 = Increment(x=w391) -> (x+1=w390:dbl)
                  n381 = for {
                    N: w390 -> [_]
                    tunnel: w392 -> [w404]
                    tunnel: [w400] -> w389
                    i -> [w403]
                    n382 = local read "frames"() -> (w402:dbl[])
                    n383 = Add(x=w404, y=w403) -> (x+y=w401:dbl)
                    n384 = Insert Into Array(array=w402, new element=w401) -> (w400:dbl[])  [unwired: 1 in]
                    n385 = local write "frames"(w400) -> ()
                  }
                }
                n386 = local write "Playback\nscore"(w361) -> ()
                n387 = property on="Search score" class="Slide (strict)"("Visible"=w361) -> ()  [unwired: 2 in, 2 out]
                n388 = Array Size(array=w356) -> (size(s)=w353:i32)
                n389 = property on="play back" class="Slide (strict)"("Scale.Maximum"=w353, "Scale.Minimum"=w355, "Maximum"=w353) -> ()  [unwired: 2 in, 2 out]
                n390 = property on="writing" class="Slide (strict)"("Scale.Maximum"=w353, "Scale.Minimum"=w355) -> ()  [unwired: 2 in, 2 out]
                "frames" <- w357
              }
            }
            n391 = local write "edit video"(w98) -> ()
          }
          frame #1 {
            w638 = 0.0 ("X Scale.Range:Minimum")
            w677 = i16 1 ("width (-)")
            w819 = dbl[] [0.0, 0.0, 0.0, 0.0, 0.0, 0.0, 0.0, 0.0] ("array")
            w805 = string[] ["Winners", "Errors"] ("W/E1")
            w786 = string[] ["Fore hand", "Back hand", "Over head", "", "Straight", "Cross", "", "Smash", "Defence", "Drive/Tap", "Lob", "Drop", "Chop", "Clear", "Net"] ("Player 2")
            w780 = "" ("new element/subarray")
            w779 = "" ("new element/subarray")
            w732 = 9 ("index")
            w727 = 9 ("index")
            n392 = local read "edited\nevents"() -> (w698:dbl[][])
            n393 = local read "filedata in"() -> (w704:dbl[][])
            n394 = Array Size(array=w698) -> (size(s)=w710:i32[])
            n395 = Index Array(array=w704, index (col)=0 ("disabled index (col)")) -> (element=w706:dbl[])  [unwired: 1 in]
            n396 = Index Array(array=w698, index (col)=0 ("disabled index (col)")) -> (element=w703:dbl[])  [unwired: 1 in]
            n397 = Index Array(array=w710, index=0) -> (element=w708:i32)
            n398 = local read "Compare"() -> (w654:bool)
            n399 = for {
              N: w708 -> [_]
              tunnel: w706 -> [w847]
              tunnel: w703 -> [w846] mode=indexing
              tunnel: [w843] -> w696 mode=indexing
              i -> [w848]
              n400 = Search 1D Array(1D array=w847, element=w846, start index (0)=w848) -> (index of element=w844:i32)
              n401 = local read "filedata in"() -> (w845:dbl[][])
              n402 = Index Array(array=w845, index (row)=w844) -> (element=w843:dbl[])  [unwired: 1 in]
            }
            n403 = case shown="\"4\"" "display\nselection" {
              tunnel: [w833 w834 w835 w836] -> w697
              tunnel: w696 -> [_ w834 _ _]
              frame "1", Default {
                n404 = local read "filedata in"() -> (w833:dbl[][])
              }
              frame "2" {
              }
              frame "3" {
                n405 = local read "save1_data"() -> (w835:dbl[][])
              }
              frame "4" {
                n406 = local read "save2_data"() -> (w836:dbl[][])
              }
            }
            n407 = case shown="\"4\"" "2" {
              tunnel: [w826 w827 w828] -> w686
              frame "1", Default {
                n408 = local read "game"() -> (w826:i32[][])
              }
              frame "3" {
                n409 = local read "save1"() -> (w827:i32[][])
              }
              frame "4" {
                n410 = local read "save2"() -> (w828:i32[][])
              }
            }
            n411 = case shown="\"1\", Default" "1" {
              tunnel: [w829 w830 w831] -> w690
              frame "1", Default {
                n412 = local read "game"() -> (w829:i32[][])
              }
              frame "3" {
                n413 = local read "save1"() -> (w830:i32[][])
              }
              frame "4" {
                n414 = local read "save2"() -> (w831:i32[][])
              }
            }
            n415 = case shown="True" w654 {
              frame False {
                w820 = u8 0 ("Disabled")
                n416 = local read "Percentage"() -> (w821:bool)
                n417 = local write "Percentage"(w821) -> ()
                n418 = local read "display\nselection"() -> (w822:string)
                n419 = local write "display\nselection"(w822) -> ()
                n420 = property on="display\nselection" class="CmbBox"("Disabled"=w820) -> ()  [unwired: 2 in, 2 out]
                n421 = property on="Percentage" class="Bool (strict)"("Disabled"=w820) -> ()  [unwired: 2 in, 2 out]
              }
              frame True {
                w823 = u8 2 ("Disabled")
                n422 = local read "1"() -> (w825:string)
                n423 = local write "display\nselection"(w825) -> ()
                n424 = property on="display\nselection" class="CmbBox"("Disabled"=w823) -> ()  [unwired: 2 in, 2 out]
                n425 = property on="Percentage" class="Bool (strict)"("Disabled"=w823) -> ()  [unwired: 2 in, 2 out]
                n426 = local write "Percentage"(TRUE ("t")) -> ()
              }
            }
            n427 = Index Array(array=w686, index (row) #1=0 ("index (row)"), index (row) #2=1 ("index (row)")) -> (element #1=w684:i32[], element #2=w682:i32[])  [unwired: 2 in]
            n428 = Index Array(array=w690, index (row) #1=0 ("index (row)"), index (row) #2=1 ("index (row)")) -> (element #1=w685:i32[], element #2=w683:i32[])  [unwired: 2 in]
            n429 = Index Array(array=w697, index (col) #1=37 ("disabled index (col)"), index (col) #2=38 ("index (col)")) -> (element #1=w717:dbl[], element #2=w714:dbl[])  [unwired: 2 in]
            n430 = for {
              N: 22 -> [_]
              tunnel: w697 -> [w883]
              tunnel: w717 -> [w882]
              tunnel: w714 -> [w881]
              tunnel: [w879] -> w715 mode=indexing
              tunnel: [w878] -> w716 mode=indexing
              i -> [w876]
              n431 = Increment(x=w876) -> (x+1=w877:i32)
              n432 = Index Array(array=w883, index (col)=w877) -> (element=w880:dbl[])  [unwired: 1 in]
              n433 = And(x=w882, y=w880) -> (x .and. y?=w879:i32[])
              n434 = And(x=w881, y=w880) -> (x .and. y?=w878:i32[])
            }
            n435 = Divide(x=w685, y=w684) -> (x/y=w679:dbl[])
            n436 = Divide(x=w683, y=w682) -> (x/y=w678:dbl[])
            n437 = Index Array(array=w697, index (col) #1=23 ("disabled index (col)"), index (col) #2=25 ("index (col)"), index (col) #3=24 ("index (col)"), index (col) #4=26 ("index (col)")) -> (element #1=w788:dbl[], element #2=w793:dbl[], element #3=w794:dbl[], element #4=w792:dbl[])  [unwired: 4 in]
            n438 = Multiply(x=w678, y=100.0 ("new element/subarray")) -> (x*y=w673:dbl[])
            n439 = Multiply(x=100.0 ("new element/subarray"), y=w679) -> (x*y=w676:dbl[])
            n440 = Add Array Elements(numeric array=w788) -> (sum=w808:dbl)
            n441 = Add Array Elements(numeric array=w794) -> (sum=w807:dbl)
            n442 = local read "comp_p1 2"() -> (w652:dbl[])
            n443 = Split 1D Array(array=w676, index=22) -> (first subarray=→"comp_p1":dbl[], second subarray=→"comp_p1 2":dbl[])
            n444 = Split 1D Array(array=w673, index=22) -> (first subarray=→"comp_p2":dbl[], second subarray=→"comp_p2 2":dbl[])
            n445 = local read "Compare"() -> (w664:bool)
            n446 = local read "comp_p2 2"() -> (w660:dbl[])
            n447 = Add Array Elements(numeric array=w792) -> (sum=w806:dbl)
            n448 = Add Array Elements(numeric array=w793) -> (sum=w809:dbl)
            n449 = local read "Compare"() -> (w661:bool)
            n450 = Build Array(w808, w809) -> (w663:dbl[])
            n451 = Build Array(w807, w806) -> (w653:dbl[])
            n452 = Transpose 2D Array(2D array=w715) -> (transposed array=w726:i32[][])
            n453 = Transpose 2D Array(2D array=w716) -> (transposed array=w725:i32[][])
            n454 = Select(t=w652, s=w664, f=w663) -> (s? t:f=w662:dbl[])
            n455 = Select(t=w660, s=w661, f=w653) -> (s? t:f=w659:dbl[])
            n456 = for {
              N: 22 -> [_]
              tunnel: w726 -> [w875]
              tunnel: w725 -> [w874]
              tunnel: [w871] -> w611 mode=indexing
              tunnel: [w870] -> w599 mode=indexing
              i -> [w873]
              n457 = Index Array(array=w875, index (col)=w873) -> (element=w872:i32[])  [unwired: 1 in]
              n458 = Index Array(array=w874, index (col)=w873) -> (element=w869:i32[])  [unwired: 1 in]
              n459 = Add Array Elements(numeric array=w872) -> (sum=w871:i32)
              n460 = Add Array Elements(numeric array=w869) -> (sum=w870:i32)
            }
            n461 = Number To Decimal String(number=w662, width (-)=w677) -> (decimal integer string=→"W1/E1":string[])
            n462 = Number To Decimal String(number=w659, width (-)=w677) -> (decimal integer string=→"W2/E2":string[])
            n463 = Split 1D Array(array=w611, index=w727) -> (first subarray=w728:i32[], second subarray=w598:i32[])
            n464 = Split 1D Array(array=w599, index=w732) -> (first subarray=w731:i32[], second subarray=w736:i32[])
            n465 = Insert Into Array(array=w611, new element=w652) -> (w702:i32[])  [unwired: 1 in]
            n466 = Insert Into Array(array=w599, new element=w653) -> (w701:i32[])  [unwired: 1 in]
            n467 = Add Array Elements(numeric array=w731) -> (sum=w730:i32)
            n468 = Add Array Elements(numeric array=w728) -> (sum=w729:i32)
            n469 = Build Array(w702, w701) -> (w694:i32[][])
            n470 = Index Array(array=w736, index #1=3 ("index"), index #2=4 ("index")) -> (element #1=w724:i32, element #2=w723:i32)
            n471 = Index Array(array=w598, index #1=3 ("index"), index #2=4 ("index")) -> (element #1=w733:i32, element #2=w734:i32)
            n472 = for {
              N: w727 -> [_]
              tunnel: w728 -> [w868] mode=indexing
              tunnel: w729 -> [w867]
              tunnel: [w864] -> w757 mode=indexing
              n473 = Divide(x=w868, y=w867) -> (x/y=w866:dbl)
              n474 = Multiply(x=w866, y=100.0) -> (x*y=w864:dbl)
            }
            n475 = Add(x=w724, y=w723) -> (x+y=w735:i32)
            n476 = for {
              N: w732 -> [_]
              tunnel: w731 -> [w863] mode=indexing
              tunnel: w730 -> [w862]
              tunnel: [w859] -> w656 mode=indexing
              n477 = Divide(x=w863, y=w862) -> (x/y=w861:dbl)
              n478 = Multiply(x=w861, y=100.0) -> (x*y=w859:dbl)
            }
            n479 = Add(x=w733, y=w734) -> (x+y=w737:i32)
            n480 = case shown="\"1\"" "display\nselection" {
              tunnel: w694 -> [_ w832 _]
              frame "0", Default {
              }
              frame "1" {
                "game" <- w832
              }
              frame "2" {
              }
            }
            n481 = case shown="False" "save2" {
              tunnel: w694 -> [_ w839]
              tunnel: w697 -> [_ w837]
              frame False {
              }
              frame True {
                n482 = local write "save2"(FALSE ("save2")) -> ()
                "save2" <- w839
                "save2_data" <- w837
              }
            }
            n483 = case shown="False" "save1" {
              tunnel: w694 -> [_ w842]
              tunnel: w697 -> [_ w840]
              frame False {
              }
              frame True {
                n484 = local write "save1"(FALSE ("save1")) -> ()
                "save1" <- w842
                "save1_data" <- w840
              }
            }
            n485 = for {
              tunnel: w736 -> [w858] mode=indexing
              tunnel: w735 -> [w857]
              tunnel: [w854] -> w759 mode=indexing
              n486 = Divide(x=w858, y=w857) -> (x/y=w856:dbl)
              n487 = Multiply(x=w856, y=100.0) -> (x*y=w854:dbl)
            }
            n488 = for {
              tunnel: w598 -> [w853] mode=indexing
              tunnel: w737 -> [w852]
              tunnel: [w849] -> w758 mode=indexing
              n489 = Divide(x=w853, y=w852) -> (x/y=w851:dbl)
              n490 = Multiply(x=w851, y=100.0) -> (x*y=w849:dbl)
            }
            n491 = local read "comp_p2"() -> (w668:dbl[])
            n492 = local read "Compare"() -> (w667:bool)
            n493 = local read "comp_p1"() -> (w669:dbl[])
            n494 = Insert Into Array(array=w656, new element=w759) -> (w655:dbl[])  [unwired: 1 in]
            n495 = Insert Into Array(array=w757, new element=w758) -> (w657:dbl[])  [unwired: 1 in]
            n496 = Select(t=w668, s=w667, f=w655) -> (s? t:f=w620:dbl[])
            n497 = Select(t=w669, s="Compare", f=w657) -> (s? t:f=w615:dbl[])
            n498 = local read "Percentage"() -> (w784:bool)
            n499 = local read "Percentage"() -> (w785:bool)
            n500 = Split 1D Array(array=w620, index=9) -> (second subarray=w765:dbl[])  [unwired: 1 out]
            n501 = Number To Fractional String(number=w620, precision (6)=i16 0) -> (F-format string=w619:string[])  [unwired: 2 in]
            n502 = Split 1D Array(array=w599, index=9) -> (second subarray=w768:i32[])  [unwired: 1 out]
            n503 = Split 1D Array(array=w615, index=9) -> (second subarray=w764:dbl[])  [unwired: 1 out]
            n504 = Number To Fractional String(number=w615, precision (6)=i16 0) -> (F-format string=w612:string[])  [unwired: 2 in]
            n505 = Split 1D Array(array=w611, index=9) -> (second subarray=w762:i32[])  [unwired: 1 out]
            n506 = local read "Percentage"() -> (w772:bool)
            n507 = Number To Fractional String(number=w611, precision (6)=i16 0) -> (F-format string=w613:string[])  [unwired: 2 in]
            n508 = Number To Decimal String(number=w762, width (-)=i16 1 ("precision (6)")) -> (decimal integer string=w771:string[])
            n509 = Number To Fractional String(number=w599, precision (6)=i16 0) -> (F-format string=w617:string[])  [unwired: 2 in]
            n510 = Number To Fractional String(number=w764, precision (6)=i16 0) -> (F-format string=w770:string[])  [unwired: 2 in]
            n511 = Number To Decimal String(number=w768, width (-)=i16 1 ("precision (6)")) -> (decimal integer string=w774:string[])
            n512 = Number To Fractional String(number=w765, precision (6)=i16 0) -> (F-format string=w773:string[])  [unwired: 2 in]
            n513 = Select(t=w612, s=w785, f=w613) -> (s? t:f=w601:string[])
            n514 = Select(t=w770, s="Percentage", f=w771) -> (s? t:f=w637:string[])
            n515 = call "Search NaN_Inf (SubVI).vi"("in"=w601) -> ("out"=w600:string[])
            n516 = Select(t=w773, s=w772, f=w774) -> (s? t:f=w634:string[])
            n517 = Select(t=w619, s=w784, f=w617) -> (s? t:f=w621:string[])
            n518 = call "Search NaN_Inf (SubVI).vi"("in"=w637) -> ("out"=w636:string[])
            n519 = call "Search NaN_Inf (SubVI).vi"("in"=w621) -> ("out"=w624:string[])
            n520 = call "Search NaN_Inf (SubVI).vi"("in"=w634) -> ("out"=w635:string[])
            n521 = Insert Into Array(array=w636, index=3, new element=w779) -> (w777:string[])
            n522 = Index Array(array=w600, index #1=0 ("index"), index #2=1 ("index"), index #3=2 ("index"), index #4=3 ("index"), index #5=4 ("index"), index #6=5 ("index"), index #7=6 ("index"), index #8=7 ("index"), index #9=8 ("index")) -> (element #1=→"p1 1":string, element #2=→"p1 2":string, element #3=→"p1 3":string, element #4=→"p1 4":string, element #5=→"p1 5":string, element #6=→"p1 6":string, element #7=→"p1 7":string, element #8=→"p1 8":string, element #9=→"p1 9":string)
            n523 = Insert Into Array(array=w635, index=3, new element=w780) -> (w782:string[])
            n524 = Insert Into Array(array=w777, index=6, new element=w779) -> (w795:string[])
            n525 = Index Array(array=w624, index #1=0 ("index"), index #2=1 ("index"), index #3=2 ("index"), index #4=3 ("index"), index #5=4 ("index"), index #6=5 ("index"), index #7=6 ("index"), index #8=7 ("index"), index #9=8 ("index")) -> (element #1=→"p2 17":string, element #2=→"p2 16":string, element #3=→"p2 12":string, element #4=→"p2 13":string, element #5=→"p2 15":string, element #6=→"p2 14":string, element #7=→"p2 10":string, element #8=→"p2 11":string, element #9=→"p2 9":string)
            n526 = Insert Into Array(array=w782, index=6, new element=w780) -> (w803:string[])
            n527 = Split 1D Array(array=w795, index=6) -> (first subarray=→"player1_2":string[], second subarray=w798:string[])
            n528 = Split 1D Array(array=w803, index=6) -> (first subarray=→"player2_2":string[], second subarray=w801:string[])
            n529 = Delete From Array(array=w798, index=0) -> (array with subset deleted=w639:string[])  [unwired: 1 in, 1 out]
            "player1 2" <- w639
            n530 = Delete From Array(array=w801, index=0) -> (array with subset deleted=w640:string[])  [unwired: 1 in, 1 out]
            "player2 2" <- w640
            n531 = Fract/Exp String To Number(string=w639) -> (number=w633:dbl[])  [unwired: 3 in, 1 out]
            n532 = Fract/Exp String To Number(string=w640) -> (number=w632:dbl[])  [unwired: 3 in, 1 out]
            n533 = Array Max & Min(array=w633) -> (max value=w648:dbl)  [unwired: 3 out]
            n534 = Array Max & Min(array=w632) -> (max value=w647:dbl)  [unwired: 3 out]
            n535 = Interleave 1D Arrays(w819, w633) -> (w651:dbl[])
            n536 = Insert Into Array(array=w651, new element=0.0 ("new element/subarray")) -> (w813:dbl[])  [unwired: 1 in]
            n537 = Max & Min(x=w648, y=w647) -> (max(x,y)=w642:dbl)  [unwired: 1 out]
            n538 = Interleave 1D Arrays(w819, w632) -> (w649:dbl[])
            n539 = Bundle(w813, "array"=dbl[] [1.0, 2.0, 3.0, 4.0, 5.0, 6.0, 7.0, 8.0, 9.0, 10.0, 11.0, 12.0, 13.0, 14.0, 15.0, 16.0, 17.0]) -> (→"P1graph":cluster{dbl[], "array":dbl[]})  [unwired: 1 in]
            n540 = Equal?(x=w642, y=inf) -> (x = y?=w644:bool)
            n541 = Insert Into Array(array=w649, new element=0.0 ("new element/subarray")) -> (w814:dbl[])  [unwired: 1 in]
            n542 = Select(t=100.0, s=w644, f=w642) -> (s? t:f=w641:dbl)
            n543 = Bundle(w814, "array"=dbl[] [1.0, 2.0, 3.0, 4.0, 5.0, 6.0, 7.0, 8.0, 9.0, 10.0, 11.0, 12.0, 13.0, 14.0, 15.0, 16.0, 17.0]) -> (→"P2graph":cluster{dbl[], "array":dbl[]})  [unwired: 1 in]
            n544 = property on="P2graph" class="XYGraph (strict)"("XScale.Maximum"=w641, "XScale.Minimum"=w638) -> ()  [unwired: 2 in, 2 out]
            n545 = property on="P1graph" class="XYGraph (strict)"("XScale.Maximum"=w641, "XScale.Minimum"=w638) -> ()  [unwired: 2 in, 2 out]
            "Player 1" <- w786
            "Player 1_2" <- w786
            "Player 2_2" <- w786
            "Player 2" <- w786
            "W/E1" <- w805
            "W/E2" <- w805
          }
        }
        n546 = case shown="True" "Play" {
          frame False {
            w931 = 0 ("play back")
            n547 = property on="Compare" class="Bool (strict)"("DisabledEnum"=w931) -> ()  [unwired: 2 in, 2 out]
            n548 = property on="Percentage" class="Bool (strict)"("DisabledEnum"=w931) -> ()  [unwired: 2 in, 2 out]
            n549 = property on="save2" class="Bool (strict)"("DisabledEnum"=w931) -> ()  [unwired: 2 in, 2 out]
            n550 = property on="save1" class="Bool (strict)"("DisabledEnum"=w931) -> ()  [unwired: 2 in, 2 out]
            n551 = property on="display\nselection" class="CmbBox"("DisabledEnum"=w931) -> ()  [unwired: 2 in, 2 out]
          }
          frame True {
            w944 = T4 4 items=["Grayscale (U8)", "Grayscale (I16)", "Grayscale (SGL)", "Complex (CSG)", "RGB (U32)", "HSL (U32)", "RGB (U64)"] ("Image Type")
            n552 = local read "Vid file"() -> (w932:path)
            n553 = local write "play back"(0 ("play back")) -> ()
            n554 = local write "Play"(FALSE ("Play")) -> ()
            n555 = call "IMAQ AVI Open"("AVI Path"=w932) -> ("error out"=w935:errorcluster, "Avi Refnum"=w937:T5)  [unwired: 9 in]
            n556 = call "IMAQ Create"("Image Name"="Disp1", "Image Type"=w944) -> ("New Image"=w943:T1, "error out"=w942:errorcluster)  [unwired: 3 in]
            n557 = call "IMAQ AVI Get Info"("error in (no error)"=w935, "Avi Refnum"=w937) -> ("Avi Refnum (duplicate)"=w936:T5, "Frame Data"=w934:T6)  [unwired: 5 in, 3 out]
            n558 = Unbundle By Name(w934) -> ("framesPerSecond"=w933:u32)
            n559 = while {
              tunnel: w936 -> [w965]
              tunnel: w943 -> [w967]
              tunnel: w942 -> [w966]
              tunnel: [FALSE ("Play")] -> w938
              tunnel: [w952] -> w940
              tunnel: w933 -> [w948]
              stop <- w958 stop-if-true
              w946 = 2 ("play back")
              n560 = local read "frames"() -> (w963:dbl[])
              n561 = Increment(x="play back") -> (x+1=w954:i32)
              n562 = Index Array(array=w963, index=w954) -> (element=w962:dbl)
              n563 = Array Max & Min(array=w963) -> (max value=w961:dbl)  [unwired: 3 out]
              n564 = Divide(x=w954, y=25.0) -> (x/y=→"Numeric":dbl)
              n565 = Divide(x=1000.0, y="Playback Speed") -> (x/y=w949:dbl)
              n566 = local write "play back"(w954) -> ()
              n567 = Divide(x=w949, y=w948) -> (x/y=w947:dbl)
              n568 = Wait (ms)(milliseconds to wait=w947) -> ()  [unwired: 1 out]
              n569 = Equal?(x=w962, y=w961) -> (x = y?=w960:bool)
              n570 = call "IMAQ AVI Read Frame"("error in (no error)"=w966, "Frame Number"=w962, "Image"=w967, "Avi Refnum"=w965) -> ("Image Out"=→"DISP":T1, "Avi Refnum (duplicate)"=w952:T5)  [unwired: 4 in, 2 out]
              n571 = Or(x=w960, y="stop 2") -> (x .or. y?=w958:bool)
              n572 = while {
                stop <- w969 continue-if-true
                n573 = local read "stop 2"() -> (w968:bool)
                n574 = Not(x=w968) -> (.not. x?=w971:bool)
                n575 = And(x=w971, y="pause") -> (x .and. y?=w969:bool)
              }
              n576 = property on="Compare" class="Bool (strict)"("DisabledEnum"=w946) -> ()  [unwired: 2 in, 2 out]
              n577 = property on="Percentage" class="Bool (strict)"("DisabledEnum"=w946) -> ()  [unwired: 2 in, 2 out]
              n578 = property on="save2" class="Bool (strict)"("DisabledEnum"=w946) -> ()  [unwired: 2 in, 2 out]
              n579 = property on="save1" class="Bool (strict)"("DisabledEnum"=w946) -> ()  [unwired: 2 in, 2 out]
              n580 = property on="display\nselection" class="CmbBox"("DisabledEnum"=w946) -> ()  [unwired: 2 in, 2 out]
            }
            n581 = local write "stop 2"(w938) -> ()
            n582 = call "IMAQ AVI Close"("Avi Refnum"=w940) -> ()  [unwired: 10 in, 1 out]
          }
        }
        n583 = case shown="True" "write file" {
          frame False {
          }
          frame True {
            n584 = local write "writing"(0 ("writing")) -> ()
            n585 = call <vilib>:"Get File Extension.vi"("file"="Write VI") -> ("filename without extension"=w885:string)  [unwired: 7 in, 3 out]
            n586 = Strip Path(path="Write VI") -> (stripped path=w886:path)  [unwired: 1 out]
            n587 = call <vilib>:"Check if File or Folder Exists.vi"("path"=w886) -> ("file or folder exists?"=w888:bool)  [unwired: 8 in, 2 out]
            n588 = case shown="True" w888 {
              tunnel: w886 -> [_ w900]
              tunnel: w885 -> [_ w899]
              frame False {
                w890 = FALSE ("Visible")
                n589 = local write "Write VI"(path "" ("Write VI")) -> ()
                n590 = local write "write file"(w890) -> ()
                n591 = property on="writing" class="Slide (strict)"("Visible"=w890) -> ()  [unwired: 2 in, 2 out]
              }
              frame True {
                w915 = T4 4 items=["Grayscale (U8)", "Grayscale (I16)", "Grayscale (SGL)", "Complex (CSG)", "RGB (U32)", "HSL (U32)", "RGB (U64)"] ("Image Type")
                n592 = local read "Vid file"() -> (w916:path)
                n593 = Path To String(path=w900) -> (string=w902:string)
                n594 = property on="writing" class="Slide (strict)"("Visible"=TRUE) -> ()  [unwired: 2 in, 2 out]
                n595 = call "IMAQ AVI Open"("AVI Path"=w916) -> ("error out"=w896:errorcluster, "Avi Refnum"=w897:T5)  [unwired: 9 in]
                n596 = Concatenate Strings(w902, "\\" ("string"), w899, ".avi" ("string")) -> (w901:string)
                n597 = call "IMAQ AVI Get Info"("error in (no error)"=w896, "Avi Refnum"=w897) -> ("Avi Refnum (duplicate)"=w898:T5, "Frame Data"=w895:T6)  [unwired: 5 in, 3 out]
                n598 = Unbundle By Name(w895) -> ("framesPerSecond"=w894:u32)
                n599 = String To Path(string=w901) -> (path=w891:path)
                n600 = local read "frames"() -> (w893:dbl[])
                n601 = local write "Write VI"(w891) -> ()
                n602 = call "IMAQ Create"("Image Name"="write", "Image Type"=w915) -> ("New Image"=w913:T1, "error out"=w912:errorcluster)  [unwired: 3 in]
                n603 = call "IMAQ AVI Create"("Compression Filter"="Microsoft Video 1", "Frames Per Second"=w894, "AVI Path"=w891) -> ("Avi Refnum"=w917:T5)  [unwired: 7 in, 1 out]
                n604 = Array Size(array=w893) -> (size(s)=w918:i32)
                n605 = for {
                  N: w918 -> [_]
                  tunnel: w917 -> [w927]
                  tunnel: w898 -> [w920]
                  tunnel: w913 -> [w929]
                  tunnel: w912 -> [w928]
                  tunnel: [w921] -> w911
                  tunnel: [FALSE ("Play")] -> w910
                  tunnel: ["Writing complete" ("message")] -> w909
                  tunnel: [w919] -> w908
                  tunnel: [w923] -> w907
                  tunnel: w893 -> [w922] mode=indexing
                  i -> [w925]
                  n606 = call "IMAQ AVI Read Frame"("error in (no error)"=w928, "Frame Number"=w922, "Image"=w929, "Avi Refnum"=w920) -> ("error out"=w930:errorcluster, "Image Out"=w923:T1, "Avi Refnum (duplicate)"=w919:T5)  [unwired: 4 in, 1 out]
                  n607 = call "IMAQ AVI Write Frame"("error in (no error)"=w930, "Image"=w923, "Avi Refnum"=w927) -> ("Avi Refnum (duplicate)"=w921:T5)  [unwired: 7 in, 1 out]
                  "writing" <- w925
                }
                n608 = local write "write file"(w910) -> ()
                n609 = property on="writing" class="Slide (strict)"("Visible"=w910) -> ()  [unwired: 2 in, 2 out]
                n610 = call "IMAQ AVI Close"("Avi Refnum"=w911) -> ()  [unwired: 10 in, 1 out]
                n611 = call "IMAQ AVI Close"("Avi Refnum"=w908) -> ("error out"=w906:errorcluster)  [unwired: 10 in]
                n612 = One Button Dialog(message=w909) -> ()  [unwired: 1 in, 1 out]
                n613 = call "IMAQ Dispose"("Image"=w907, "error in (no error)"=w906) -> ()  [unwired: 4 in, 1 out]
              }
            }
          }
        }
        n614 = case shown="True" "REPORT" {
          frame False {
          }
          frame True {
            w97 = TRUE ("open new instance (false)")
            n615 = Automation Open(Automation Refnum="Word._Application", 9:w97) -> (Automation Refnum=w88:refnum<k7>, error out=w89:errorcluster)  [unwired: 2 in]
            n616 = Current VI's Path() -> (path=w95:path)
            n617 = property class="_Application"(reference=w88, error in=w89, "Visible"=w97) -> (reference out=w90:refnum<k7>, error out=w91:errorcluster)
            n618 = Strip Path(path=w95) -> (stripped path=w96:path)  [unwired: 1 out]
            n619 = Build Path(base path=w96, name or relative path="BStAT report.doc") -> (appended path=w82:path)
            n620 = One Button Dialog(message="Right-click on the white strip on the LEFT of the data area to copy the data") -> ()  [unwired: 1 in, 1 out]
            n621 = local write "REPORT"(FALSE ("REPORT")) -> ()
            n622 = property class="_Application"(reference=w90, error in=w91) -> (error out=w93:errorcluster, "Documents"=w92:refnum<k7>)  [unwired: 1 out]
            n623 = invoke class="Documents" method="Open"(reference=w92, error in=w93, "FileName"=w82, "ReadOnly"=TRUE, "Visible"=TRUE) -> ()  [unwired: 14 in, 19 out]
          }
        }
      }
      frame True {
        w972 = u32 0 ("S_frame")
        n624 = local write "Drag control"(w972) -> ()
        n625 = local write "START"(FALSE ("START")) -> ()
        n626 = stacked-sequence {
          frame #0 {
            w990 = 0 ("p2code")
            w998 = T4 4 items=["Grayscale (U8)", "Grayscale (I16)", "Grayscale (SGL)", "Complex (CSG)", "RGB (U32)", "HSL (U32)", "RGB (U64)"] ("Image Type")
            n627 = local read "Video file"() -> (w974:path)
            n628 = call "IMAQ Create"("Image Name"="setup", "Image Type"=w998) -> ("New Image"=w996:T1, "error out"=w994:errorcluster)  [unwired: 3 in]
            n629 = call "IMAQ AVI Open"("AVI Path"=w974) -> ("Avi Refnum"=w999:T5)  [unwired: 9 in, 1 out]
            n630 = local read "Video file"() -> (w981:path)
            n631 = call "IMAQ AVI Get Info"("Avi Refnum"=w999) -> ("Number of Frames"=w1000:u32, "Avi Refnum (duplicate)"=w992:T5, "Frame Data"=w986:T6)  [unwired: 6 in, 2 out]
            n632 = while {
              tunnel: w992 -> [w1012]
              tunnel: w996 -> [w1011]
              tunnel: w994 -> [w1010]
              tunnel: [FALSE ("Visible")] -> w987
              tunnel: [w1007] -> w995
              tunnel: [w1006] -> w991
              stop <- "Start Coding" stop-if-true
              w1005 = TRUE ("Visible")
              n633 = call "IMAQ AVI Read Frame"("error in (no error)"=w1010, "Frame Number"="Drag control", "Image"=w1011, "Avi Refnum"=w1012) -> ("Image Out"=→"Video":T1, "Avi Refnum (duplicate)"=w1007:T5)  [unwired: 4 in, 2 out]
              n634 = case shown="False" "F_Fr" {
                tunnel: "Drag control" -> [_ w1014]
                frame False {
                }
                frame True {
                  n635 = local write "F_frame"(w1014) -> ()
                  n636 = local write "F_Fr"(FALSE ("F_Fr")) -> ()
                }
              }
              n637 = case shown="False" "S_Fr" {
                tunnel: "Drag control" -> [_ w1016]
                frame False {
                }
                frame True {
                  n638 = local write "S_frame"(w1016) -> ()
                  n639 = local write "S_Fr"(FALSE ("S_Fr")) -> ()
                }
              }
              n640 = property on="Drag control" class="Slide (strict)"("Visible"=w1005) -> ()  [unwired: 2 in, 2 out]
              n641 = property on="S_frame" class="DigNum (strict)"("Visible"=w1005) -> ()  [unwired: 2 in, 2 out]
              n642 = property on="Start Coding" class="Bool (strict)"("Visible"=w1005) -> ()  [unwired: 2 in, 2 out]
              n643 = property on="S_Fr" class="Bool (strict)"("Visible"=w1005) -> ()  [unwired: 2 in, 2 out]
              n644 = property on="F_frame" class="DigNum (strict)"("Visible"=w1005) -> ()  [unwired: 2 in, 2 out]
              n645 = property on="F_Fr" class="Bool (strict)"("Visible"=w1005) -> ()  [unwired: 2 in, 2 out]
              n646 = local read "S_frame"() -> (w1006:u32)
            }
            n647 = Decrement(x=w1000) -> (x-1=w989:u32)
            n648 = local read "Save data"() -> (w975:path)
            n649 = Path To String(path=w981) -> (string=w980:string)
            n650 = property on="Drag control" class="Slide (strict)"("Scale.Maximum"=w989, "Scale.Minimum"=0.0 ("Scale.Range:Minimum")) -> ()  [unwired: 2 in, 2 out]
            n651 = Path To String(path=w975) -> (string=w984:string)
            n652 = call <vilib>:"Search and Replace Pattern.vi"("string"=w980, "regular expression (\"\")"=".avi" ("regular expression (\"\")"), "replace string (\"\")"=".xls" ("replace string (\"\")")) -> ("result string"=w978:string)  [unwired: 2 in, 1 out]
            n653 = Empty String/Path?(string/path=w984) -> (empty?=w979:bool)
            n654 = String To Path(string=w978) -> (path=w976:path)
            n655 = Unbundle By Name(w986) -> ("framesPerSecond"=→"framesPerSecond":u32)
            n656 = One Button Dialog(message="Please Select the start and end points\nof the video for coding ") -> ()  [unwired: 1 in, 1 out]
            n657 = Select(t=w976, s=w979, f=w975) -> (s? t:f=w977:path)
            n658 = local write "Save data"(w977) -> ()
            n659 = call "IMAQ AVI Close"("Avi Refnum"=w995) -> ()  [unwired: 10 in, 1 out]
            n660 = local write "Progress..."(w991) -> ()
            n661 = local write "p2code"(w990) -> ()
            n662 = local write "p1code"(w990) -> ()
            n663 = local write "Start Coding"(w987) -> ()
            n664 = property on="S_frame" class="DigNum (strict)"("Visible"=w987) -> ()  [unwired: 2 in, 2 out]
            n665 = property on="F_frame" class="DigNum (strict)"("Visible"=w987) -> ()  [unwired: 2 in, 2 out]
            n666 = property on="Start Coding" class="Bool (strict)"("Visible"=w987) -> ()  [unwired: 2 in, 2 out]
            n667 = property on="S_Fr" class="Bool (strict)"("Visible"=w987) -> ()  [unwired: 2 in, 2 out]
            n668 = property on="F_Fr" class="Bool (strict)"("Visible"=w987) -> ()  [unwired: 2 in, 2 out]
          }
          frame #1 {
            w1026 = "\r"
            w1022 = TRUE ("Visible")
            w1020 = TRUE ("Visible")
            w1041 = T4 4 items=["Grayscale (U8)", "Grayscale (I16)", "Grayscale (SGL)", "Complex (CSG)", "RGB (U32)", "HSL (U32)", "RGB (U64)"] ("Image Type")
            n669 = local read "Video file"() -> (w1030:path)
            n670 = call "IMAQ Create"("Image Name"="code", "Image Type"=w1041) -> ("New Image"=w1040:T1, "error out"=w1039:errorcluster)  [unwired: 3 in]
            n671 = call "IMAQ AVI Open"("AVI Path"=w1030) -> ("Avi Refnum"=w1038:T5)  [unwired: 9 in, 1 out]
            n672 = while {
              tunnel: w1040 -> [w1073]
              tunnel: w1039 -> [w1072]
              tunnel: w1038 -> [w1078]
              tunnel: [FALSE] -> w1023
              tunnel: [w1080] -> w1019
              tunnel: [w1077] -> w1024
              tunnel: [w1065] -> w1018
              tunnel: [w1064] -> w1017
              stop <- w1058 stop-if-true
              n673 = case shown="True" "switch sides" {
                frame False {
                }
                frame True {
                  n674 = stacked-sequence {
                    frame #0 {
                      n675 = property on="W2" class="Bool (strict)"() -> ("Position"=w1099:T7)  [unwired: 2 in, 2 out]
                      n676 = property on="W1" class="Bool (strict)"() -> ("Position"=w1100:T7)  [unwired: 2 in, 2 out]
                      n677 = property on="E2" class="Bool (strict)"() -> ("Position"=w1101:T7)  [unwired: 2 in, 2 out]
                      n678 = property on="E1" class="Bool (strict)"() -> ("Position"=w1102:T7)  [unwired: 2 in, 2 out]
                      n679 = property on="P2" class="DigNum (strict)"() -> ("Position"=w1103:T7)  [unwired: 2 in, 2 out]
                      n680 = property on="P1" class="DigNum (strict)"() -> ("Position"=w1104:T7)  [unwired: 2 in, 2 out]
                      n681 = property on="Pause 1" class="Bool (strict)"() -> ("Position"=w1105:T7)  [unwired: 2 in, 2 out]
                      n682 = property on="Pause 2" class="Bool (strict)"() -> ("Position"=w1106:T7)  [unwired: 2 in, 2 out]
                      n683 = property on="S2" class="Bool (strict)"() -> ("Position"=w1098:T7)  [unwired: 2 in, 2 out]
                      n684 = property on="S1" class="Bool (strict)"() -> ("Position"=w1097:T7)  [unwired: 2 in, 2 out]
                      n685 = Bundle("Position"=w1099, "Position"=w1100, "Position"=w1101, "Position"=w1102, "Position"=w1103, "Position"=w1104, "Position"=w1105, "Position"=w1106, "Position"=w1098, "Position"=w1097) -> (w1107:T8)  [unwired: 1 in]
                      n686 = local write "switch sides"(FALSE ("switch sides")) -> ()
                      n687 = Unbundle(w1107) -> ("Position"=w1108:T7, "Position"=w1109:T7, "Position"=w1110:T7, "Position"=w1111:T7, "Position"=w1112:T7, "Position"=w1113:T7, "Position"=w1114:T7, "Position"=w1115:T7, "Position"=w1096:T7, "Position"=w1095:T7)
                      n688 = property on="S1" class="Bool (strict)"("Position"=w1096) -> ()  [unwired: 2 in, 2 out]
                      n689 = property on="S2" class="Bool (strict)"("Position"=w1095) -> ()  [unwired: 2 in, 2 out]
                      n690 = property on="W1" class="Bool (strict)"("Position"=w1108) -> ()  [unwired: 2 in, 2 out]
                      n691 = property on="W2" class="Bool (strict)"("Position"=w1109) -> ()  [unwired: 2 in, 2 out]
                      n692 = property on="E1" class="Bool (strict)"("Position"=w1110) -> ()  [unwired: 2 in, 2 out]
                      n693 = property on="E2" class="Bool (strict)"("Position"=w1111) -> ()  [unwired: 2 in, 2 out]
                      n694 = property on="P1" class="DigNum (strict)"("Position"=w1112) -> ()  [unwired: 2 in, 2 out]
                      n695 = property on="P2" class="DigNum (strict)"("Position"=w1113) -> ()  [unwired: 2 in, 2 out]
                      n696 = property on="Pause 2" class="Bool (strict)"("Position"=w1114) -> ()  [unwired: 2 in, 2 out]
                      n697 = property on="Pause 1" class="Bool (strict)"("Position"=w1115) -> ()  [unwired: 2 in, 2 out]
                    }
                    frame #1 {
                      n698 = property on="TL 2" class="Bool (strict)"() -> ("Position"=w1117:T7)  [unwired: 2 in, 2 out]
                      n699 = property on="TL 3" class="Bool (strict)"() -> ("Position"=w1118:T7)  [unwired: 2 in, 2 out]
                      n700 = property on="ML 2" class="Bool (strict)"() -> ("Position"=w1119:T7)  [unwired: 2 in, 2 out]
                      n701 = property on="ML 3" class="Bool (strict)"() -> ("Position"=w1120:T7)  [unwired: 2 in, 2 out]
                      n702 = property on="BL 2" class="Bool (strict)"() -> ("Position"=w1121:T7)  [unwired: 2 in, 2 out]
                      n703 = property on="BL 3" class="Bool (strict)"() -> ("Position"=w1122:T7)  [unwired: 2 in, 2 out]
                      n704 = Bundle("Position"=w1117, "Position"=w1118, "Position"=w1119, "Position"=w1120, "Position"=w1121, "Position"=w1122) -> (w1116:T9)  [unwired: 1 in]
                      n705 = Unbundle(w1116) -> ("Position"=w1123:T7, "Position"=w1124:T7, "Position"=w1125:T7, "Position"=w1126:T7, "Position"=w1127:T7, "Position"=w1128:T7)
                      n706 = property on="TL 3" class="Bool (strict)"("Position"=w1123) -> ()  [unwired: 2 in, 2 out]
                      n707 = property on="TL 2" class="Bool (strict)"("Position"=w1124) -> ()  [unwired: 2 in, 2 out]
                      n708 = property on="ML 3" class="Bool (strict)"("Position"=w1125) -> ()  [unwired: 2 in, 2 out]
                      n709 = property on="ML 2" class="Bool (strict)"("Position"=w1126) -> ()  [unwired: 2 in, 2 out]
                      n710 = property on="BL 3" class="Bool (strict)"("Position"=w1127) -> ()  [unwired: 2 in, 2 out]
                      n711 = property on="BL 2" class="Bool (strict)"("Position"=w1128) -> ()  [unwired: 2 in, 2 out]
                    }
                    frame #2 {
                      n712 = property on="BC 2" class="Bool (strict)"() -> ("Position"=w1130:T7)  [unwired: 2 in, 2 out]
                      n713 = property on="TC 3" class="Bool (strict)"() -> ("Position"=w1131:T7)  [unwired: 2 in, 2 out]
                      n714 = property on="TC 2" class="Bool (strict)"() -> ("Position"=w1132:T7)  [unwired: 2 in, 2 out]
                      n715 = property on="MC 3" class="Bool (strict)"() -> ("Position"=w1133:T7)  [unwired: 2 in, 2 out]
                      n716 = property on="MC 2" class="Bool (strict)"() -> ("Position"=w1134:T7)  [unwired: 2 in, 2 out]
                      n717 = property on="BC 3" class="Bool (strict)"() -> ("Position"=w1135:T7)  [unwired: 2 in, 2 out]
                      n718 = Bundle("Position"=w1130, "Position"=w1131, "Position"=w1132, "Position"=w1133, "Position"=w1134, "Position"=w1135) -> (w1129:T9)  [unwired: 1 in]
                      n719 = Unbundle(w1129) -> ("Position"=w1136:T7, "Position"=w1137:T7, "Position"=w1138:T7, "Position"=w1139:T7, "Position"=w1140:T7, "Position"=w1141:T7)
                      n720 = property on="BC 3" class="Bool (strict)"("Position"=w1136) -> ()  [unwired: 2 in, 2 out]
                      n721 = property on="TC 2" class="Bool (strict)"("Position"=w1137) -> ()  [unwired: 2 in, 2 out]
                      n722 = property on="TC 3" class="Bool (strict)"("Position"=w1138) -> ()  [unwired: 2 in, 2 out]
                      n723 = property on="MC 2" class="Bool (strict)"("Position"=w1139) -> ()  [unwired: 2 in, 2 out]
                      n724 = property on="MC 3" class="Bool (strict)"("Position"=w1140) -> ()  [unwired: 2 in, 2 out]
                      n725 = property on="BC 2" class="Bool (strict)"("Position"=w1141) -> ()  [unwired: 2 in, 2 out]
                    }
                    frame #3 {
                      n726 = property on="BR 3" class="Bool (strict)"() -> ("Position"=w1143:T7)  [unwired: 2 in, 2 out]
                      n727 = property on="MR  3" class="Bool (strict)"() -> ("Position"=w1144:T7)  [unwired: 2 in, 2 out]
                      n728 = property on="TR 3" class="Bool (strict)"() -> ("Position"=w1145:T7)  [unwired: 2 in, 2 out]
                      n729 = property on="TR 2" class="Bool (strict)"() -> ("Position"=w1146:T7)  [unwired: 2 in, 2 out]
                      n730 = property on="MR  2" class="Bool (strict)"() -> ("Position"=w1147:T7)  [unwired: 2 in, 2 out]
                      n731 = property on="BR 2" class="Bool (strict)"() -> ("Position"=w1148:T7)  [unwired: 2 in, 2 out]
                      n732 = Bundle("Position"=w1143, "Position"=w1144, "Position"=w1145, "Position"=w1146, "Position"=w1147, "Position"=w1148) -> (w1142:T9)  [unwired: 1 in]
                      n733 = Unbundle(w1142) -> ("Position"=w1149:T7, "Position"=w1150:T7, "Position"=w1151:T7, "Position"=w1152:T7, "Position"=w1153:T7, "Position"=w1154:T7)
                      n734 = property on="BR 2" class="Bool (strict)"("Position"=w1149) -> ()  [unwired: 2 in, 2 out]
                      n735 = property on="MR  2" class="Bool (strict)"("Position"=w1150) -> ()  [unwired: 2 in, 2 out]
                      n736 = property on="TR 2" class="Bool (strict)"("Position"=w1151) -> ()  [unwired: 2 in, 2 out]
                      n737 = property on="TR 3" class="Bool (strict)"("Position"=w1152) -> ()  [unwired: 2 in, 2 out]
                      n738 = property on="MR  3" class="Bool (strict)"("Position"=w1153) -> ()  [unwired: 2 in, 2 out]
                      n739 = property on="BR 3" class="Bool (strict)"("Position"=w1154) -> ()  [unwired: 2 in, 2 out]
                    }
                  }
                }
              }
              n740 = Increment(x="Progress...") -> (x+1=w1079:i32)
              n741 = call "IMAQ AVI Read Frame"("error in (no error)"=w1072, "Frame Number"=w1079, "Image"=w1073, "Avi Refnum"=w1078) -> ("Image Out"=w1057:T1)  [unwired: 4 in, 3 out]
              n742 = local write "Video"(w1057) -> ()
              n743 = local read "F_frame"() -> (w1083:u32)
              n744 = Add(x=9, y=w1079) -> (x+y=w1082:i32)
              n745 = local read "framesPerSecond"() -> (w1056:u32)
              n746 = Less Or Equal?(x=w1083, y=w1082) -> (x <= y?=w1062:bool)
              n747 = Select(t=w1082, s="fast forward", f=w1079) -> (s? t:f=w1061:i32)
              n748 = Select(t="Progress...", s=w1062, f=w1061) -> (s? t:f=w1059:i32)
              n749 = Divide(x=1000.0, y="playback speed") -> (x/y=w1086:dbl)
              n750 = local write "Progress..."(w1059) -> ()
              n751 = Divide(x=w1086, y=w1056) -> (x/y=w1055:dbl)
              n752 = Wait (ms)(milliseconds to wait=w1055) -> ()  [unwired: 1 out]
              n753 = Compound Arithmetic op=OR("Pause 1", "Pause 2", "Pause 3") -> (w1081:bool)
              n754 = case shown="True" w1081 {
                tunnel: w1079 -> [w1167 w1247]
                tunnel: [w1166 w1232] -> w1080
                tunnel: w1079 -> [_ w1250]
                tunnel: w1078 -> [w1164 w1249]
                tunnel: [w1164 w1246] -> w1077
                tunnel: "Pause 1" -> [_ w1245]
                tunnel: "Pause 2" -> [_ w1244]
                tunnel: w1055 -> [_ w1240]
                frame False {
                  n755 = local read "W1"() -> (w1163:bool)
                  n756 = local read "W2"() -> (w1161:bool)
                  n757 = local read "E1"() -> (w1162:bool)
                  n758 = local read "E2"() -> (w1160:bool)
                  n759 = Or(x=w1163, y=w1162) -> (x .or. y?=w1159:bool)
                  n760 = Or(x=w1161, y=w1160) -> (x .or. y?=w1158:bool)
                  n761 = Boolean To (0,1)(Boolean=w1159) -> (0, 1=w1156:i16)
                  n762 = Select(t=2.0, s=w1158, f=w1156) -> (s? t:f=w1155:dbl)
                  n763 = case shown="1" w1155 {
                    tunnel: w1167 -> [_ _ _]
                    tunnel: [w1170 w1199 w1202] -> w1166
                    tunnel: [FALSE FALSE FALSE] -> w1165
                    frame 0, Default {
                      w1168 = FALSE ("4 6")
                      n764 = local write "1 6"(w1168) -> ()
                      n765 = local write "2 6"(w1168) -> ()
                      n766 = local write "3 6"(w1168) -> ()
                      n767 = local write "4 6"(w1168) -> ()
                      n768 = local write "5 6"(w1168) -> ()
                      n769 = local write "6 6"(w1168) -> ()
                      n770 = local write "7 6"(w1168) -> ()
                      n771 = local write "8 6"(w1168) -> ()
                      n772 = local write "1 5"(w1168) -> ()
                      n773 = local write "2 5"(w1168) -> ()
                      n774 = local write "3 5"(w1168) -> ()
                      n775 = local write "4 5"(w1168) -> ()
                      n776 = local write "5 5"(w1168) -> ()
                      n777 = local write "6 5"(w1168) -> ()
                      n778 = local write "7 5"(w1168) -> ()
                      n779 = local write "8 5"(w1168) -> ()
                      n780 = local write "1 4"(w1168) -> ()
                      n781 = local write "2 4"(w1168) -> ()
                      n782 = local write "3 4"(w1168) -> ()
                      n783 = local write "4 4"(w1168) -> ()
                      n784 = local write "5 4"(w1168) -> ()
                      n785 = local write "6 4"(w1168) -> ()
                      n786 = local write "7 4"(w1168) -> ()
                      n787 = local write "8 4"(w1168) -> ()
                      n788 = local write "1 3"(w1168) -> ()
                      n789 = local write "2 3"(w1168) -> ()
                      n790 = local write "3 3"(w1168) -> ()
                      n791 = local write "4 3"(w1168) -> ()
                      n792 = local write "5 3"(w1168) -> ()
                      n793 = local write "6 3"(w1168) -> ()
                      n794 = local write "7 3"(w1168) -> ()
                      n795 = local write "8 3"(w1168) -> ()
                      n796 = local write "1 2"(w1168) -> ()
                      n797 = local write "2 2"(w1168) -> ()
                      n798 = local write "3 2"(w1168) -> ()
                      n799 = local write "4 2"(w1168) -> ()
                      n800 = local write "5 2"(w1168) -> ()
                      n801 = local write "6 2"(w1168) -> ()
                      n802 = local write "7 2"(w1168) -> ()
                      n803 = local write "8 2"(w1168) -> ()
                      n804 = local write "1"(w1168) -> ()
                      n805 = local write "2"(w1168) -> ()
                      n806 = local write "3"(w1168) -> ()
                      n807 = local write "4"(w1168) -> ()
                      n808 = local write "5"(w1168) -> ()
                      n809 = local write "6"(w1168) -> ()
                      n810 = local write "7"(w1168) -> ()
                      n811 = local write "8"(w1168) -> ()
                      n812 = local write "BL 3"(w1168) -> ()
                      n813 = local write "BL 2"(w1168) -> ()
                      n814 = local write "BR 2"(w1168) -> ()
                      n815 = local write "BR 3"(w1168) -> ()
                      n816 = local write "W1"(w1168) -> ()
                      n817 = local write "W2"(w1168) -> ()
                      n818 = local write "E1"(w1168) -> ()
                      n819 = local write "E2"(w1168) -> ()
                      n820 = local write "BC 3"(w1168) -> ()
                      n821 = local write "BC 2"(w1168) -> ()
                      n822 = local write "TL 3"(w1168) -> ()
                      n823 = local write "TL 2"(w1168) -> ()
                      n824 = local write "TR 2"(w1168) -> ()
                      n825 = local write "TR 3"(w1168) -> ()
                      n826 = local write "S1"(w1168) -> ()
                      n827 = local write "S2"(w1168) -> ()
                      n828 = local write "1"(w1168) -> ()
                      n829 = local write "2"(w1168) -> ()
                      n830 = local write "3"(w1168) -> ()
                      n831 = local write "4"(w1168) -> ()
                      n832 = local write "TC 2"(w1168) -> ()
                      n833 = local write "TC 3"(w1168) -> ()
                      n834 = local write "ML 3"(w1168) -> ()
                      n835 = local write "ML 2"(w1168) -> ()
                      n836 = local write "MR  2"(w1168) -> ()
                      n837 = local write "MR  3"(w1168) -> ()
                      n838 = local write "MC 2"(w1168) -> ()
                      n839 = local write "MC 3"(w1168) -> ()
                      n840 = local read "coding"() -> (w1170:i32[][])
                    }
                    frame 1 {
                      n841 = local read "W1"() -> (w1193:bool)
                      n842 = local read "W2"() -> (w1194:bool)
                      n843 = local read "E1"() -> (w1195:bool)
                      n844 = local read "E2"() -> (w1196:bool)
                      n845 = Boolean To (0,1)(Boolean=w1193) -> (0, 1=w1185:i16)
                      n846 = Boolean To (0,1)(Boolean=w1194) -> (0, 1=w1184:i16)
                      n847 = Boolean To (0,1)(Boolean=w1195) -> (0, 1=w1179:i16)
                      n848 = Boolean To (0,1)(Boolean=w1196) -> (0, 1=w1178:i16)
                      n849 = Or(x=w1193, y=w1196) -> (x .or. y?=w1192:bool)
                      n850 = Or(x=w1194, y=w1195) -> (x .or. y?=w1191:bool)
                      n851 = local read "P2"() -> (w1171:i32)
                      n852 = local read "P1"() -> (w1197:i32)
                      n853 = Increment(x=w1197) -> (x+1=w1190:i32)
                      n854 = Increment(x=w1171) -> (x+1=w1189:i32)
                      n855 = Select(t=w1189, s=w1191, f=w1171) -> (s? t:f=w1172:i32)
                      n856 = Select(t=w1190, s=w1192, f=w1197) -> (s? t:f=w1174:i32)
                      n857 = Boolean To (0,1)(Boolean=w1192) -> (0, 1=w1177:i16)
                      n858 = Boolean To (0,1)(Boolean=w1191) -> (0, 1=w1176:i16)
                      n859 = local write "P1"(w1174) -> ()
                      n860 = local write "P2"(w1172) -> ()
                      n861 = local read "p1code"() -> (w1187:i32)
                      n862 = local read "coding"() -> (w1198:i32[][])
                      n863 = Replace Array Subset(array=w1198, new element #1=w1185, index (row) #1=w1187, index (col) #1=23 ("disabled index (col)"), new element #2=w1184, index (row) #2=w1187, index (col) #2=24 ("disabled index (col)"), new element #3=w1179, index (row) #3=w1187, index (col) #3=25 ("disabled index (col)"), new element #4=w1178, index (row) #4=w1187, index (col) #4=26 ("disabled index (col)"), new element #5=w1177, index (row) #5=w1187, index (col) #5=27 ("disabled index (col)"), new element #6=w1176, index (row) #6=w1187, index (col) #6=28 ("disabled index (col)"), new element #7=w1174, index (row) #7=w1187, index (col) #7=29 ("disabled index (col)"), new element #8=w1172, index (row) #8=w1187, index (col) #8=30 ("disabled index (col)")) -> (w1199:i32[][])
                      n864 = local write "coding"(w1199) -> ()
                    }
                    frame 2 {
                      n865 = local read "W1"() -> (w1225:bool)
                      n866 = local read "W2"() -> (w1226:bool)
                      n867 = local read "E1"() -> (w1227:bool)
                      n868 = local read "E2"() -> (w1228:bool)
                      n869 = Boolean To (0,1)(Boolean=w1225) -> (0, 1=w1218:i16)
                      n870 = Boolean To (0,1)(Boolean=w1226) -> (0, 1=w1217:i16)
                      n871 = Boolean To (0,1)(Boolean=w1227) -> (0, 1=w1212:i16)
                      n872 = Boolean To (0,1)(Boolean=w1228) -> (0, 1=w1211:i16)
                      n873 = Or(x=w1225, y=w1228) -> (x .or. y?=w1224:bool)
                      n874 = Or(x=w1226, y=w1227) -> (x .or. y?=w1223:bool)
                      n875 = local read "P2"() -> (w1201:i32)
                      n876 = local read "P1"() -> (w1229:i32)
                      n877 = Increment(x=w1229) -> (x+1=w1222:i32)
                      n878 = Increment(x=w1201) -> (x+1=w1221:i32)
                      n879 = Select(t=w1221, s=w1223, f=w1201) -> (s? t:f=w1205:i32)
                      n880 = Select(t=w1222, s=w1224, f=w1229) -> (s? t:f=w1207:i32)
                      n881 = Boolean To (0,1)(Boolean=w1224) -> (0, 1=w1210:i16)
                      n882 = Boolean To (0,1)(Boolean=w1223) -> (0, 1=w1209:i16)
                      n883 = local write "P1"(w1207) -> ()
                      n884 = local write "P2"(w1205) -> ()
                      n885 = local read "p2code"() -> (w1203:i32)
                      n886 = local read "coding"() -> (w1230:i32[][])
                      n887 = Replace Array Subset(array=w1230, new element #1=w1218, index (row) #1=w1203, index (col) #1=23 ("disabled index (col)"), new element #2=w1217, index (row) #2=w1203, index (col) #2=24 ("disabled index (col)"), new element #3=w1212, index (row) #3=w1203, index (col) #3=25 ("disabled index (col)"), new element #4=w1211, index (row) #4=w1203, index (col) #4=26 ("disabled index (col)"), new element #5=w1210, index (row) #5=w1203, index (col) #5=27 ("disabled index (col)"), new element #6=w1209, index (row) #6=w1203, index (col) #6=28 ("disabled index (col)"), new element #7=w1207, index (row) #7=w1203, index (col) #7=29 ("disabled index (col)"), new element #8=w1205, index (row) #8=w1203, index (col) #8=30 ("disabled index (col)")) -> (w1202:i32[][])
                      n888 = local write "coding"(w1202) -> ()
                    }
                  }
                  n889 = local write "W1"(w1165) -> ()
                  n890 = local write "W2"(w1165) -> ()
                  n891 = local write "E1"(w1165) -> ()
                  n892 = local write "E2"(w1165) -> ()
                }
                frame True {
                  n893 = stacked-sequence {
                    tunnel: [_ w1333 _ _ _ _ _ _] -> w1248
                    tunnel: [_ w1332 _ _ _ _ _ _] -> w1287
                    tunnel: [_ w1331 _ _ _ _ _ _] -> w1286
                    tunnel: [_ w1330 _ _ _ _ _ _] -> w1285
                    tunnel: [_ w1329 _ _ _ _ _ _] -> w1284
                    tunnel: [_ w1328 _ _ _ _ _ _] -> w1283
                    tunnel: [_ w1327 _ _ _ _ _ _] -> w1282
                    tunnel: [_ w1326 _ _ _ _ _ _] -> w1276
                    tunnel: [_ w1325 _ _ _ _ _ _] -> w1281
                    tunnel: [_ _ _ w1403 _ _ _ _] -> w1280
                    tunnel: [_ _ _ w1402 _ _ _ _] -> w1279
                    tunnel: [_ _ _ w1400 _ _ _ _] -> w1278
                    tunnel: [_ _ _ _ w1500 _ _ _] -> w1277
                    tunnel: [_ _ _ _ w1497 _ _ _] -> w1275
                    tunnel: [_ _ _ _ w1464 _ _ _] -> w1274
                    tunnel: [_ _ _ _ w1463 _ _ _] -> w1273
                    tunnel: [_ _ _ _ w1462 _ _ _] -> w1272
                    tunnel: [_ _ _ _ w1461 _ _ _] -> w1271
                    tunnel: [_ _ _ _ w1460 _ _ _] -> w1270
                    tunnel: [_ _ _ _ w1459 _ _ _] -> w1269
                    tunnel: [_ _ _ _ w1458 _ _ _] -> w1268
                    tunnel: [_ _ _ _ w1457 _ _ _] -> w1267
                    tunnel: [_ _ _ _ _ _ w1585 _] -> w1266
                    tunnel: [_ _ _ _ _ _ w1585 _] -> w1265
                    tunnel: [_ _ _ _ _ _ w1585 _] -> w1264
                    tunnel: [_ _ _ _ _ _ w1585 _] -> w1263
                    tunnel: [_ _ _ _ _ _ w1585 _] -> w1262
                    tunnel: [_ _ _ _ _ _ w1585 _] -> w1261
                    tunnel: [_ _ _ _ _ _ w1585 _] -> w1260
                    tunnel: [_ _ _ _ _ _ w1585 _] -> w1259
                    tunnel: [_ _ _ _ _ _ w1591 _] -> w1258
                    tunnel: [_ _ _ _ _ _ w1590 _] -> w1257
                    tunnel: [_ _ _ _ _ _ w1589 _] -> w1256
                    tunnel: [_ _ _ _ _ _ w1588 _] -> w1255
                    tunnel: [_ _ _ _ _ _ w1587 _] -> w1254
                    tunnel: [_ _ _ _ _ _ w1586 _] -> w1253
                    tunnel: [_ _ w1371 _ _ _ _ _] -> w1252
                    tunnel: [_ _ w1370 _ _ _ _ _] -> w1251
                    tunnel: w1250 -> [w1296 _ _ _ _ _ _ _]
                    tunnel: w1249 -> [w1295 _ _ _ _ _ _ _]
                    tunnel: [w1294 _ _ _ _ _ _ _] -> w1246
                    tunnel: [_ _ _ _ _ _ _ w1598] -> w1233
                    tunnel: w1245 -> [_ _ w1369 _ _ _ _ _]
                    tunnel: w1244 -> [_ _ w1368 _ _ _ _ _]
                    tunnel: w1240 -> [w1289 _ _ _ _ _ _ _]
                    tunnel: [w1288 _ _ _ _ _ _ _] -> w1231
                    frame #0 {
                      w1292 = T4 4 items=["Grayscale (U8)", "Grayscale (I16)", "Grayscale (SGL)", "Complex (CSG)", "RGB (U32)", "HSL (U32)", "RGB (U64)"] ("Image Type")
                      n894 = while {
                        tunnel: [FALSE] -> w1293
                        stop <- w1318 continue-if-true
                        n895 = local read "Pause 3"() -> (w1315:bool)
                        n896 = local read "Pause 1"() -> (w1316:bool)
                        n897 = local read "Pause 2"() -> (w1319:bool)
                        n898 = local read "coding"() -> (w1310:i32[][])
                        n899 = Compound Arithmetic op=OR(w1315, w1316, w1319) -> (w1318:bool)
                        n900 = Index Array(array=w1310, index (col)=0 ("disabled index (col)")) -> (element=w1313:i32[])  [unwired: 1 in]
                        n901 = Array Max & Min(array=w1313) -> (max value=w1312:i32, max index (indices)=w1309:i32)  [unwired: 2 out]
                        n902 = Wait (ms)(milliseconds to wait=10.0 ("Delay Time (s)")) -> ()  [unwired: 1 out]
                        n903 = case shown="True" "UNDO" {
                          selector: "UNDO" -> [w1320 _]
                          tunnel: w1310 -> [_ w1324]
                          tunnel: w1309 -> [_ w1323]
                          tunnel: [w1320 FALSE] -> w1308
                          frame False {
                          }
                          frame True {
                            n904 = Delete From Array(array=w1324, index (row)=w1323) -> (array with subset deleted=w1322:i32[][])  [unwired: 2 in, 1 out]
                            n905 = local write "coding"(w1322) -> ()
                          }
                        }
                        n906 = local write "Last coded"(w1312) -> ()
                        n907 = local write "UNDO"(w1308) -> ()
                      }
                      n908 = call "IMAQ Create"("Image Name"="code3", "Image Type"=w1292) -> ("New Image"=w1288:T1, "error out"=w1290:errorcluster)  [unwired: 3 in]
                      n909 = for {
                        N: 25 -> [_]
                        tunnel: w1296 -> [w1305]
                        tunnel: w1295 -> [w1303]
                        tunnel: w1290 -> [w1302]
                        tunnel: w1288 -> [w1301]
                        tunnel: [w1300] -> w1294
                        tunnel: w1289 -> [w1299]
                        i -> [w1306]
                        n910 = Add(x=w1306, y=w1305) -> (x+y=w1304:i32)
                        n911 = call "IMAQ AVI Read Frame"("error in (no error)"=w1302, "Frame Number"=w1304, "Image"=w1301, "Avi Refnum"=w1303) -> ("Image Out"=w1298:T1, "Avi Refnum (duplicate)"=w1300:T5)  [unwired: 4 in, 2 out]
                        n912 = local write "Video"(w1298) -> ()
                        n913 = Wait (ms)(milliseconds to wait=w1299) -> ()  [unwired: 1 out]
                      }
                      n914 = local write "Pause 1"(w1293) -> ()
                      n915 = local write "Pause 2"(w1293) -> ()
                      n916 = local write "Pause 3"(w1293) -> ()
                      n917 = local write "UNDO"(w1293) -> ()
                    }
                    frame #1 {
                      n918 = Or(x="TC 2", y="TC 3") -> (x .or. y?=w1341:bool)
                      n919 = Or(x="ML 3", y="ML 2") -> (x .or. y?=w1339:bool)
                      n920 = Or(x="MR  2", y="MR  3") -> (x .or. y?=w1337:bool)
                      n921 = Or(x="BC 3", y="BC 2") -> (x .or. y?=w1335:bool)
                      n922 = Boolean To (0,1)(Boolean=w1341) -> (0, 1=w1332:i16)
                      n923 = Boolean To (0,1)(Boolean=w1339) -> (0, 1=w1330:i16)
                      n924 = Boolean To (0,1)(Boolean=w1337) -> (0, 1=w1328:i16)
                      n925 = Boolean To (0,1)(Boolean=w1335) -> (0, 1=w1326:i16)
                      n926 = Or(x="TL 3", y="TL 2") -> (x .or. y?=w1342:bool)
                      n927 = Or(x="TR 2", y="TR 3") -> (x .or. y?=w1340:bool)
                      n928 = Or(x="MC 2", y="MC 3") -> (x .or. y?=w1338:bool)
                      n929 = Or(x="BL 3", y="BL 2") -> (x .or. y?=w1336:bool)
                      n930 = Or(x="BR 2", y="BR 3") -> (x .or. y?=w1334:bool)
                      n931 = Boolean To (0,1)(Boolean=w1342) -> (0, 1=w1333:i16)
                      n932 = Boolean To (0,1)(Boolean=w1340) -> (0, 1=w1331:i16)
                      n933 = Boolean To (0,1)(Boolean=w1338) -> (0, 1=w1329:i16)
                      n934 = Boolean To (0,1)(Boolean=w1336) -> (0, 1=w1327:i16)
                      n935 = Boolean To (0,1)(Boolean=w1334) -> (0, 1=w1325:i16)
                    }
                    frame #2 {
                      n936 = local read "S1"() -> (w1367:bool)
                      n937 = local read "S2"() -> (w1366:bool)
                      n938 = local read "MR  3"() -> (w1391:bool)
                      n939 = local read "MC 3"() -> (w1395:bool)
                      n940 = local read "TC 3"() -> (w1396:bool)
                      n941 = local read "BC 3"() -> (w1394:bool)
                      n942 = local read "ML 3"() -> (w1397:bool)
                      n943 = local read "BR 3"() -> (w1393:bool)
                      n944 = local read "TR 3"() -> (w1392:bool)
                      n945 = local read "BL 3"() -> (w1399:bool)
                      n946 = local read "TL 3"() -> (w1398:bool)
                      n947 = Or(x=w1367, y=w1366) -> (x .or. y?=w1362:bool)
                      n948 = Compound Arithmetic op=OR(w1399, w1398, w1397, w1396, w1395, w1394, w1393, w1392, w1391) -> (w1373:bool)
                      "P1 position" <- w1373
                      n949 = Or(x=w1373, y=w1369) -> (x .or. y?=w1364:bool)
                      n950 = Or(x=w1364, y=w1362) -> (x .or. y?=w1365:bool)
                      n951 = local read "coding"() -> (w1381:i32[][])
                      n952 = local read "MR  2"() -> (w1385:bool)
                      n953 = local read "MC 2"() -> (w1387:bool)
                      n954 = local read "TC 2"() -> (w1388:bool)
                      n955 = local read "BC 2"() -> (w1386:bool)
                      n956 = local read "ML 2"() -> (w1382:bool)
                      n957 = local read "TR 2"() -> (w1384:bool)
                      n958 = local read "BR 2"() -> (w1383:bool)
                      n959 = local read "BL 2"() -> (w1390:bool)
                      n960 = local read "TL 2"() -> (w1389:bool)
                      n961 = Boolean To (0,1)(Boolean=w1365) -> (0, 1=w1371:i16)
                      n962 = Array Size(array=w1381) -> (size(s)=w1380:i32[])
                      n963 = Compound Arithmetic op=OR(w1390, w1389, w1382, w1388, w1387, w1386, w1385, w1384, w1383) -> (w1372:bool)
                      "P2 position" <- w1372
                      n964 = local read "p1code"() -> (w1377:i32)
                      n965 = Index Array(array=w1380, index=0) -> (element=w1375:i32)
                      n966 = Or(x=w1372, y=w1368) -> (x .or. y?=w1363:bool)
                      n967 = Or(x=w1363, y=w1362) -> (x .or. y?=w1361:bool)
                      n968 = Select(t=w1375, s=w1365, f=w1377) -> (s? t:f=→"p1code":i32)
                      n969 = local read "p2code"() -> (w1374:i32)
                      n970 = Select(t=w1375, s=w1361, f=w1374) -> (s? t:f=→"p2code":i32)
                      n971 = Boolean To (0,1)(Boolean=w1361) -> (0, 1=w1370:i16)
                    }
                    frame #3 {
                      n972 = Build Array("1", "2", "3", "4", "5", "6", "7", "8", "1 2", "2 2", "3 2", "4 2", "5 2", "6 2", "7 2", "8 2") -> (w1424:bool[])
                      "FH" <- w1424
                      n973 = Or Array Elements(Boolean array=w1424) -> (logical OR=w1405:bool)
                      n974 = Boolean To (0,1)(Boolean=w1405) -> (0, 1=w1403:i16)
                      n975 = Build Array("1 3", "2 3", "3 3", "4 3", "5 3", "6 3", "7 3", "8 3", "1 4", "2 4", "3 4", "4 4", "5 4", "6 4", "7 4", "8 4") -> (w1407:bool[])
                      "BH" <- w1407
                      n976 = Or Array Elements(Boolean array=w1407) -> (logical OR=w1404:bool)
                      n977 = Boolean To (0,1)(Boolean=w1404) -> (0, 1=w1402:i16)
                      n978 = Build Array("1 5", "2 5", "3 5", "4 5", "5 5", "6 5", "7 5", "8 5", "1 6", "2 6", "3 6", "4 6", "5 6", "6 6", "7 6", "8 6") -> (w1406:bool[])
                      "OH" <- w1406
                      n979 = Or Array Elements(Boolean array=w1406) -> (logical OR=w1401:bool)
                      n980 = Boolean To (0,1)(Boolean=w1401) -> (0, 1=w1400:i16)
                    }
                    frame #4 {
                      w1505 = 8 ("index")
                      n981 = local read "OH"() -> (w1494:bool[])
                      n982 = local read "BH"() -> (w1495:bool[])
                      n983 = local read "FH"() -> (w1496:bool[])
                      n984 = Split 1D Array(array=w1496, index=w1505) -> (first subarray=w1492:bool[], second subarray=w1493:bool[])
                      n985 = Split 1D Array(array=w1495, index=w1505) -> (first subarray=w1504:bool[], second subarray=w1502:bool[])
                      n986 = Split 1D Array(array=w1494, index=w1505) -> (first subarray=w1503:bool[], second subarray=w1501:bool[])
                      n987 = Build Array(w1492, w1504, w1503) -> (w1491:bool[][])
                      n988 = Build Array(w1493, w1502, w1501) -> (w1490:bool[][])
                      n989 = Or Array Elements(Boolean array=w1491) -> (logical OR=w1499:bool)
                      n990 = Or Array Elements(Boolean array=w1490) -> (logical OR=w1498:bool)
                      n991 = Insert Into Array(array=w1491, new element=w1490) -> (w1489:bool[][])  [unwired: 2 in]
                      n992 = Boolean To (0,1)(Boolean=w1499) -> (0, 1=w1500:i16)
                      n993 = Boolean To (0,1)(Boolean=w1498) -> (0, 1=w1497:i16)
                      n994 = Index Array(array=w1489, index (col) #1=3 ("disabled index (col)"), index (col) #2=4 ("index (col)"), index (col) #3=2 ("index (col)"), index (col) #4=1 ("index (col)"), index (col) #5=6 ("index (col)"), index (col) #6=5 ("index (col)"), index (col) #7=0 ("index (col)"), index (col) #8=7 ("index (col)")) -> (element #1=w1479:bool[], element #2=w1471:bool[], element #3=w1470:bool[], element #4=w1469:bool[], element #5=w1468:bool[], element #6=w1467:bool[], element #7=w1466:bool[], element #8=w1465:bool[])  [unwired: 8 in]
                      n995 = Or Array Elements(Boolean array=w1479) -> (logical OR=w1480:bool)
                      n996 = Or Array Elements(Boolean array=w1470) -> (logical OR=w1476:bool)
                      n997 = Or Array Elements(Boolean array=w1468) -> (logical OR=w1475:bool)
                      n998 = Or Array Elements(Boolean array=w1466) -> (logical OR=w1472:bool)
                      n999 = Or Array Elements(Boolean array=w1471) -> (logical OR=w1478:bool)
                      n1000 = Or Array Elements(Boolean array=w1469) -> (logical OR=w1477:bool)
                      n1001 = Or Array Elements(Boolean array=w1467) -> (logical OR=w1474:bool)
                      n1002 = Or Array Elements(Boolean array=w1465) -> (logical OR=w1473:bool)
                      n1003 = Boolean To (0,1)(Boolean=w1480) -> (0, 1=w1464:i16)
                      n1004 = Boolean To (0,1)(Boolean=w1476) -> (0, 1=w1462:i16)
                      n1005 = Boolean To (0,1)(Boolean=w1475) -> (0, 1=w1460:i16)
                      n1006 = Boolean To (0,1)(Boolean=w1472) -> (0, 1=w1458:i16)
                      n1007 = Boolean To (0,1)(Boolean=w1478) -> (0, 1=w1463:i16)
                      n1008 = Boolean To (0,1)(Boolean=w1477) -> (0, 1=w1461:i16)
                      n1009 = Boolean To (0,1)(Boolean=w1474) -> (0, 1=w1459:i16)
                      n1010 = Boolean To (0,1)(Boolean=w1473) -> (0, 1=w1457:i16)
                    }
                    frame #5 {
                      n1011 = local read "P2 position"() -> (w1520:bool)
                      n1012 = local read "P1 position"() -> (w1516:bool)
                      n1013 = local read "BH"() -> (w1514:bool[])
                      n1014 = local read "OH"() -> (w1515:bool[])
                      n1015 = local read "FH"() -> (w1513:bool[])
                      n1016 = Or(x="W2", y="E2") -> (x .or. y?=w1524:bool)
                      n1017 = Or(x="W1", y="E1") -> (x .or. y?=w1521:bool)
                      n1018 = Or Array Elements(Boolean array=w1514) -> (logical OR=w1518:bool)
                      n1019 = Or Array Elements(Boolean array=w1515) -> (logical OR=w1519:bool)
                      n1020 = Or Array Elements(Boolean array=w1513) -> (logical OR=w1517:bool)
                      n1021 = Compound Arithmetic op=OR(w1516, w1517, w1518, w1519, w1520) -> (invert w1523:bool)
                      n1022 = And(x=w1523, y=w1524) -> (x .and. y?=w1525:bool)
                      n1023 = And(x=w1523, y=w1521) -> (x .and. y?=w1522:bool)
                      n1024 = Boolean To (0,1)(Boolean=w1522) -> (0, 1=w1512:i16)
                      n1025 = Select(t=2.0, s=w1525, f=w1512) -> (s? t:f=w1507:dbl)
                      n1026 = case shown="1" w1507 {
                        tunnel: [w1526 w1555 w1558] -> _
                        frame 0, Default {
                          n1027 = local read "coding"() -> (w1526:i32[][])
                        }
                        frame 1 {
                          n1028 = local read "W1"() -> (w1549:bool)
                          n1029 = local read "W2"() -> (w1550:bool)
                          n1030 = local read "P2"() -> (w1527:i32)
                          n1031 = local read "E1"() -> (w1551:bool)
                          n1032 = local read "E2"() -> (w1552:bool)
                          n1033 = local read "P1"() -> (w1553:i32)
                          n1034 = Increment(x=w1527) -> (x+1=w1545:i32)
                          n1035 = Or(x=w1550, y=w1551) -> (x .or. y?=w1547:bool)
                          n1036 = Increment(x=w1553) -> (x+1=w1546:i32)
                          n1037 = Or(x=w1549, y=w1552) -> (x .or. y?=w1548:bool)
                          n1038 = Boolean To (0,1)(Boolean=w1549) -> (0, 1=w1541:i16)
                          n1039 = Boolean To (0,1)(Boolean=w1550) -> (0, 1=w1540:i16)
                          n1040 = Boolean To (0,1)(Boolean=w1551) -> (0, 1=w1535:i16)
                          n1041 = Boolean To (0,1)(Boolean=w1552) -> (0, 1=w1534:i16)
                          n1042 = Select(t=w1545, s=w1547, f=w1527) -> (s? t:f=w1528:i32)
                          n1043 = local read "p1code"() -> (w1543:i32)
                          n1044 = local read "coding"() -> (w1554:i32[][])
                          n1045 = Select(t=w1546, s=w1548, f=w1553) -> (s? t:f=w1530:i32)
                          n1046 = Boolean To (0,1)(Boolean=w1548) -> (0, 1=w1533:i16)
                          n1047 = Boolean To (0,1)(Boolean=w1547) -> (0, 1=w1532:i16)
                          n1048 = local write "P1"(w1530) -> ()
                          n1049 = local write "P2"(w1528) -> ()
                          n1050 = Replace Array Subset(array=w1554, new element #1=w1541, index (row) #1=w1543, index (col) #1=23 ("disabled index (col)"), new element #2=w1540, index (row) #2=w1543, index (col) #2=24 ("disabled index (col)"), new element #3=w1535, index (row) #3=w1543, index (col) #3=25 ("disabled index (col)"), new element #4=w1534, index (row) #4=w1543, index (col) #4=26 ("disabled index (col)"), new element #5=w1533, index (row) #5=w1543, index (col) #5=27 ("disabled index (col)"), new element #6=w1532, index (row) #6=w1543, index (col) #6=28 ("disabled index (col)"), new element #7=w1530, index (row) #7=w1543, index (col) #7=29 ("disabled index (col)"), new element #8=w1528, index (row) #8=w1543, index (col) #8=30 ("disabled index (col)")) -> (w1555:i32[][])
                          n1051 = local write "coding"(w1555) -> ()
                        }
                        frame 2 {
                          n1052 = local read "W1"() -> (w1580:bool)
                          n1053 = local read "W2"() -> (w1581:bool)
                          n1054 = local read "E1"() -> (w1582:bool)
                          n1055 = local read "E2"() -> (w1583:bool)
                          n1056 = Increment(x="P1") -> (x+1=w1577:i32)
                          n1057 = Boolean To (0,1)(Boolean=w1580) -> (0, 1=w1573:i16)
                          n1058 = Boolean To (0,1)(Boolean=w1581) -> (0, 1=w1572:i16)
                          n1059 = Boolean To (0,1)(Boolean=w1582) -> (0, 1=w1567:i16)
                          n1060 = Boolean To (0,1)(Boolean=w1583) -> (0, 1=w1566:i16)
                          n1061 = Or(x=w1580, y=w1583) -> (x .or. y?=w1579:bool)
                          n1062 = Or(x=w1581, y=w1582) -> (x .or. y?=w1578:bool)
                          n1063 = Increment(x="P2") -> (x+1=w1576:i32)
                          n1064 = Select(t=w1576, s=w1578, f="P2") -> (s? t:f=w1560:i32)
                          n1065 = Select(t=w1577, s=w1579, f="P1") -> (s? t:f=w1562:i32)
                          n1066 = Boolean To (0,1)(Boolean=w1579) -> (0, 1=w1565:i16)
                          n1067 = Boolean To (0,1)(Boolean=w1578) -> (0, 1=w1564:i16)
                          n1068 = local read "p2code"() -> (w1559:i32)
                          n1069 = local read "coding"() -> (w1584:i32[][])
                          n1070 = local write "P1"(w1562) -> ()
                          n1071 = Replace Array Subset(array=w1584, new element #1=w1573, index (row) #1=w1559, index (col) #1=23 ("disabled index (col)"), new element #2=w1572, index (row) #2=w1559, index (col) #2=24 ("disabled index (col)"), new element #3=w1567, index (row) #3=w1559, index (col) #3=25 ("disabled index (col)"), new element #4=w1566, index (row) #4=w1559, index (col) #4=26 ("disabled index (col)"), new element #5=w1565, index (row) #5=w1559, index (col) #5=27 ("disabled index (col)"), new element #6=w1564, index (row) #6=w1559, index (col) #6=28 ("disabled index (col)"), new element #7=w1562, index (row) #7=w1559, index (col) #7=29 ("disabled index (col)"), new element #8=w1560, index (row) #8=w1559, index (col) #8=30 ("disabled index (col)")) -> (w1558:i32[][])
                          n1072 = local write "P2"(w1560) -> ()
                          n1073 = local write "coding"(w1558) -> ()
                        }
                      }
                    }
                    frame #6 {
                      w1585 = i16 0
                      n1074 = Boolean To (0,1)(Boolean="S1") -> (0, 1=w1591:i16)
                      n1075 = Boolean To (0,1)(Boolean="S2") -> (0, 1=w1590:i16)
                      n1076 = Boolean To (0,1)(Boolean="1") -> (0, 1=w1589:i16)
                      n1077 = Boolean To (0,1)(Boolean="2") -> (0, 1=w1588:i16)
                      n1078 = Boolean To (0,1)(Boolean="3") -> (0, 1=w1587:i16)
                      n1079 = Boolean To (0,1)(Boolean="4") -> (0, 1=w1586:i16)
                    }
                    frame #7 {
                      w1599 = FALSE ("4 6")
                      n1080 = local write "1 6"(w1599) -> ()
                      n1081 = local write "2 6"(w1599) -> ()
                      n1082 = local write "3 6"(w1599) -> ()
                      n1083 = local write "4 6"(w1599) -> ()
                      n1084 = local write "5 6"(w1599) -> ()
                      n1085 = local write "6 6"(w1599) -> ()
                      n1086 = local write "7 6"(w1599) -> ()
                      n1087 = local write "8 6"(w1599) -> ()
                      n1088 = local write "1 5"(w1599) -> ()
                      n1089 = local write "2 5"(w1599) -> ()
                      n1090 = local write "3 5"(w1599) -> ()
                      n1091 = local write "4 5"(w1599) -> ()
                      n1092 = local write "5 5"(w1599) -> ()
                      n1093 = local write "6 5"(w1599) -> ()
                      n1094 = local write "7 5"(w1599) -> ()
                      n1095 = local write "8 5"(w1599) -> ()
                      n1096 = local write "1 4"(w1599) -> ()
                      n1097 = local write "2 4"(w1599) -> ()
                      n1098 = local write "3 4"(w1599) -> ()
                      n1099 = local write "4 4"(w1599) -> ()
                      n1100 = local write "5 4"(w1599) -> ()
                      n1101 = local write "6 4"(w1599) -> ()
                      n1102 = local write "7 4"(w1599) -> ()
                      n1103 = local write "8 4"(w1599) -> ()
                      n1104 = local write "1 3"(w1599) -> ()
                      n1105 = local write "2 3"(w1599) -> ()
                      n1106 = local write "3 3"(w1599) -> ()
                      n1107 = local write "4 3"(w1599) -> ()
                      n1108 = local write "5 3"(w1599) -> ()
                      n1109 = local write "6 3"(w1599) -> ()
                      n1110 = local write "7 3"(w1599) -> ()
                      n1111 = local write "8 3"(w1599) -> ()
                      n1112 = local write "1 2"(w1599) -> ()
                      n1113 = local write "2 2"(w1599) -> ()
                      n1114 = local write "3 2"(w1599) -> ()
                      n1115 = local write "4 2"(w1599) -> ()
                      n1116 = local write "5 2"(w1599) -> ()
                      n1117 = local write "6 2"(w1599) -> ()
                      n1118 = local write "7 2"(w1599) -> ()
                      n1119 = local write "8 2"(w1599) -> ()
                      n1120 = local write "1"(w1599) -> ()
                      n1121 = local write "2"(w1599) -> ()
                      n1122 = local write "3"(w1599) -> ()
                      n1123 = local write "4"(w1599) -> ()
                      n1124 = local write "5"(w1599) -> ()
                      n1125 = local write "6"(w1599) -> ()
                      n1126 = local write "7"(w1599) -> ()
                      n1127 = local write "8"(w1599) -> ()
                      n1128 = local write "BL 3"(w1599) -> ()
                      n1129 = local write "BL 2"(w1599) -> ()
                      n1130 = local write "BR 2"(w1599) -> ()
                      n1131 = local write "BR 3"(w1599) -> ()
                      n1132 = local write "BC 3"(w1599) -> ()
                      n1133 = local write "BC 2"(w1599) -> ()
                      n1134 = local write "W1"(w1599) -> ()
                      n1135 = local write "W2"(w1599) -> ()
                      n1136 = local write "E1"(w1599) -> ()
                      n1137 = local write "E2"(w1599) -> ()
                      n1138 = local write "TL 3"(w1599) -> ()
                      n1139 = local write "TL 2"(w1599) -> ()
                      n1140 = local write "TR 2"(w1599) -> ()
                      n1141 = local write "TR 3"(w1599) -> ()
                      n1142 = local write "TC 2"(w1599) -> ()
                      n1143 = local write "TC 3"(w1599) -> ()
                      n1144 = local write "S1"(w1599) -> ()
                      n1145 = local write "S2"(w1599) -> ()
                      n1146 = local write "1"(w1599) -> ()
                      n1147 = local write "2"(w1599) -> ()
                      n1148 = local write "3"(w1599) -> ()
                      n1149 = local write "4"(w1599) -> ()
                      n1150 = local read "coding"() -> (w1598:i32[][])
                      n1151 = local write "ML 3"(w1599) -> ()
                      n1152 = local write "ML 2"(w1599) -> ()
                      n1153 = local write "MR  2"(w1599) -> ()
                      n1154 = local write "MR  3"(w1599) -> ()
                      n1155 = local write "MC 2"(w1599) -> ()
                      n1156 = local write "MC 3"(w1599) -> ()
                    }
                  }
                  n1157 = call "IMAQ Dispose"("Image"=w1231) -> ()  [unwired: 5 in, 1 out]
                  n1158 = Build Array(w1247, w1248, w1287, w1286, w1285, w1284, w1283, w1282, w1276, w1281, w1280, w1279, w1278, w1277, w1275, w1274, w1273, w1272, w1271, w1270, w1269, w1268, w1267, w1266, w1265, w1264, w1263, w1262, w1261, w1260, w1259, w1258, w1257, w1256, w1255, w1254, w1253, w1252, w1251) -> (w1239:i32[])
                  n1159 = Delete From Array(array=w1239, index=0) -> (array with subset deleted=w1237:i32[])  [unwired: 1 in, 1 out]
                  n1160 = Insert Into Array(array=w1233, new element=w1239) -> (w1234:i32[][])  [unwired: 2 in]
                  n1161 = Array Max & Min(array=w1237) -> (max value=w1236:i32)  [unwired: 3 out]
                  n1162 = Equal To 0?(x=w1236) -> (x = 0?=w1235:bool)
                  n1163 = Select(t=w1233, s=w1235, f=w1234) -> (s? t:f=w1232:i32[][])
                  n1164 = Index Array(array=w1232, index (col)=0 ("disabled index (col)")) -> (element=w1241:i32[])  [unwired: 1 in]
                  n1165 = Array Max & Min(array=w1241) -> (max value=→"Last coded":i32)  [unwired: 3 out]
                  n1166 = local write "coding"(w1232) -> ()
                }
              }
              n1167 = case shown="True" "Stop and save" {
                tunnel: [FALSE ("T button?") w1091] -> w1058
                frame False {
                }
                frame True {
                  n1168 = Two Button Dialog(message="You are about to stop the notation process", 2:"Stop and Save" ("Left Button Text (\"Yes\")")) -> (T button?=w1091:bool)  [unwired: 1 in]
                }
              }
              n1169 = Strip Path(path="Save data") -> (stripped path=w1068:path)  [unwired: 1 out]
              n1170 = call <vilib>:"Get File Extension.vi"("file"="Save data") -> ("filename without extension"=w1071:string)  [unwired: 7 in, 3 out]
              n1171 = Path To String(path=w1068) -> (string=w1067:string)
              n1172 = Concatenate Strings(w1067, "\\" ("string"), w1071, "(BStAT DATA).xls" ("string")) -> (w1066:string)
              n1173 = String To Path(string=w1066) -> (path=w1064:path)
              n1174 = call <vilib>:"Check if File or Folder Exists.vi"("path"=w1064) -> ("file or folder exists?"=w1065:bool)  [unwired: 8 in, 2 out]
            }
            n1175 = local read "F_frame"() -> (w1036:u32)
            n1176 = local read "S_frame"() -> (w1035:u32)
            n1177 = property on="Progress..." class="Slide (strict)"("Scale.Maximum"=w1036, "Scale.Minimum"=w1035, "Visible"=w1020) -> ()  [unwired: 2 in, 2 out]
            n1178 = Not(x=w1020) -> (.not. x?=w1021:bool)
            n1179 = property on="Drag control" class="Slide (strict)"("Visible"=w1021) -> ()  [unwired: 2 in, 2 out]
            n1180 = Path to Array of Strings(0:w1030) -> (2:w1031:string[])  [unwired: 1 out]
            n1181 = Array Size(array=w1031) -> (size(s)=w1032:i32)
            n1182 = Decrement(x=w1032) -> (x-1=w1033:i32)
            n1183 = Index Array(array=w1031, index=w1033) -> (element=w1029:string)
            n1184 = call "EVENTS(SubVI).vi"() -> ("Events"=w1027:string)  [unwired: 1 in]
            n1185 = Concatenate Strings("avi file" ("string"), w1026, w1029, w1026, w1026, w1027) -> (w1028:string)
            n1186 = call "IMAQ AVI Close"("Avi Refnum"=w1024) -> ()  [unwired: 10 in, 1 out]
            n1187 = case shown="False" w1018 {
              tunnel: w1019 -> [w1049 w1051]
              tunnel: w1028 -> [w1046 _]
              tunnel: w1017 -> [w1044 w1050]
              frame False {
                n1188 = Open/Create/Replace File(file path (use dialog)=w1044, operation (0:open)=T3."create") -> (refnum out=w1047:refnum<file>)  [unwired: 4 in, 2 out]
                n1189 = Write to Text File(file (use dialog)=w1047, text=w1046) -> (refnum out=w1043:refnum<file>)  [unwired: 2 in, 2 out]
                n1190 = Close File(refnum=w1043) -> (path=w1042:path)  [unwired: 1 in, 1 out]
                n1191 = call-poly <vilib>:"Write To Spreadsheet File.vi"("append to file? (new file:F)"=TRUE, "2D data"=w1049, "file path (dialog if empty)"=w1042) -> ()  [unwired: 5 in, 1 out]
              }
              frame True {
                n1192 = call-poly <vilib>:"Write To Spreadsheet File.vi"("append to file? (new file:F)"=TRUE, "2D data"=w1051, "file path (dialog if empty)"=w1050) -> ()  [unwired: 5 in, 1 out]
              }
            }
            n1193 = property on="playback speed" class="Slide (strict)"("Visible"=w1023) -> ()  [unwired: 2 in, 2 out]
            n1194 = property on="Progress..." class="Slide (strict)"("Visible"=w1023) -> ()  [unwired: 2 in, 2 out]
            n1195 = property on="UNDO" class="Bool (strict)"("Visible"=w1023) -> ()  [unwired: 2 in, 2 out]
            n1196 = property on="Last coded" class="DigNum (strict)"("Visible"=w1023) -> ()  [unwired: 2 in, 2 out]
            n1197 = property on="Last coded" class="DigNum (strict)"("Visible"=w1022) -> ()  [unwired: 2 in, 2 out]
            n1198 = property on="UNDO" class="Bool (strict)"("Visible"=w1022) -> ()  [unwired: 2 in, 2 out]
            n1199 = property on="playback speed" class="Slide (strict)"("Visible"=w1022) -> ()  [unwired: 2 in, 2 out]
            "coding" <- i32[][] [] ("coding")
          }
        }
        "S_frame" <- w972
        "F_frame" <- w972
      }
    }
  }
